vi "AimingBeamCodeTest.vi"() -> ()   [LabVIEW 2024]
doc: "Main VI for FLS imaging system."
uses:
  SubVI/DigitizerConfiguration/FLImDAQ.ctl
  <instrlib>/niScope/Controls/niScope trigger source.ctl
  ConfigFiles/AimingBeamVideoConfig.ctl
  <vilib>/Utility/error.llb/DialogType.ctl
  <vilib>/numeric/Random Number (Range) DBL.vi
  SubVI/GlobalVariables.vi
  <userlib>/_OpenG.lib/file/file.llb/openg_file.lvlib
  <userlib>/_OpenG.lib/time/time.llb/openg_time.lvlib
  <vilib>/Utility/miscctls.llb/LVPointTypeDef.ctl
panel:
  in  "VideoConfig":T1={"DeCon Channel"=enum."1", "Scale Bar"=FALSE, "Scale Low"=10.0, "Scale High"=200.0, "ANSI"=20.0, "Radius"=1.0, "3D?"=FALSE, "Firefly?"=FALSE, "Pentero?"=FALSE}
  out "Lifetime":dbl
  in  "MainLoopExit?":errorcluster
  out "SendLifetime?":bool
  in  "Channel":enum16{"Ch1", "Ch2", "Ch3"}(ring)
  out "Visualization PC video source":T2
  in  "Video Display":bool
  out "ML?":bool
  out "remote address":string
  out "Sync Success?":bool
  out "Disclamer":picture
  out "Calibration #":i8
  out "BG #":i8
  in  "TCP Connect":bool
  out "Help":string
  out "Run":i8 caption="Run #"
  in  "StopButton":bool caption="Stop"
  out "Aquisition Status:":bool
  in  "StartButton":bool caption="Start"
  in  "Video Source":enum32{"Camera", "FrameGrabber"}(radio)
  out "Case #":string
  out "System Hardware Connection Status":T3
  in  "Tab Control":T4(tab)
  out "Communication loop(ms)":u32
  out "FLImDAQ":T5={"Digitizer 1"="", "Digitizer 2"="", "Channel"=enum."Channel 0", "trigger source"="VAL_EXTERNAL", "trigger level"=0.5, "trigger delay"=1.35e-07, "min sample rate"=12500000000.0, "min record length"=2500, "vertical range"=1.0, "vertical offset"=-0.25, "Waveform to Avg"=2000} caption="FLIm DAQ Configuration" {"trigger delay" format="%^#.4e"; "trigger level" min=0.0 max=3.5 step=0.5 format="%.2f"; "vertical offset" format="%.4f"; "vertical range" format="%.2f"; "min sample rate" format="%#.2p"}
  out "data out(communcation loop)":string
  out "syctimer data out":string
  out "State log":string
  in  "Quit":bool
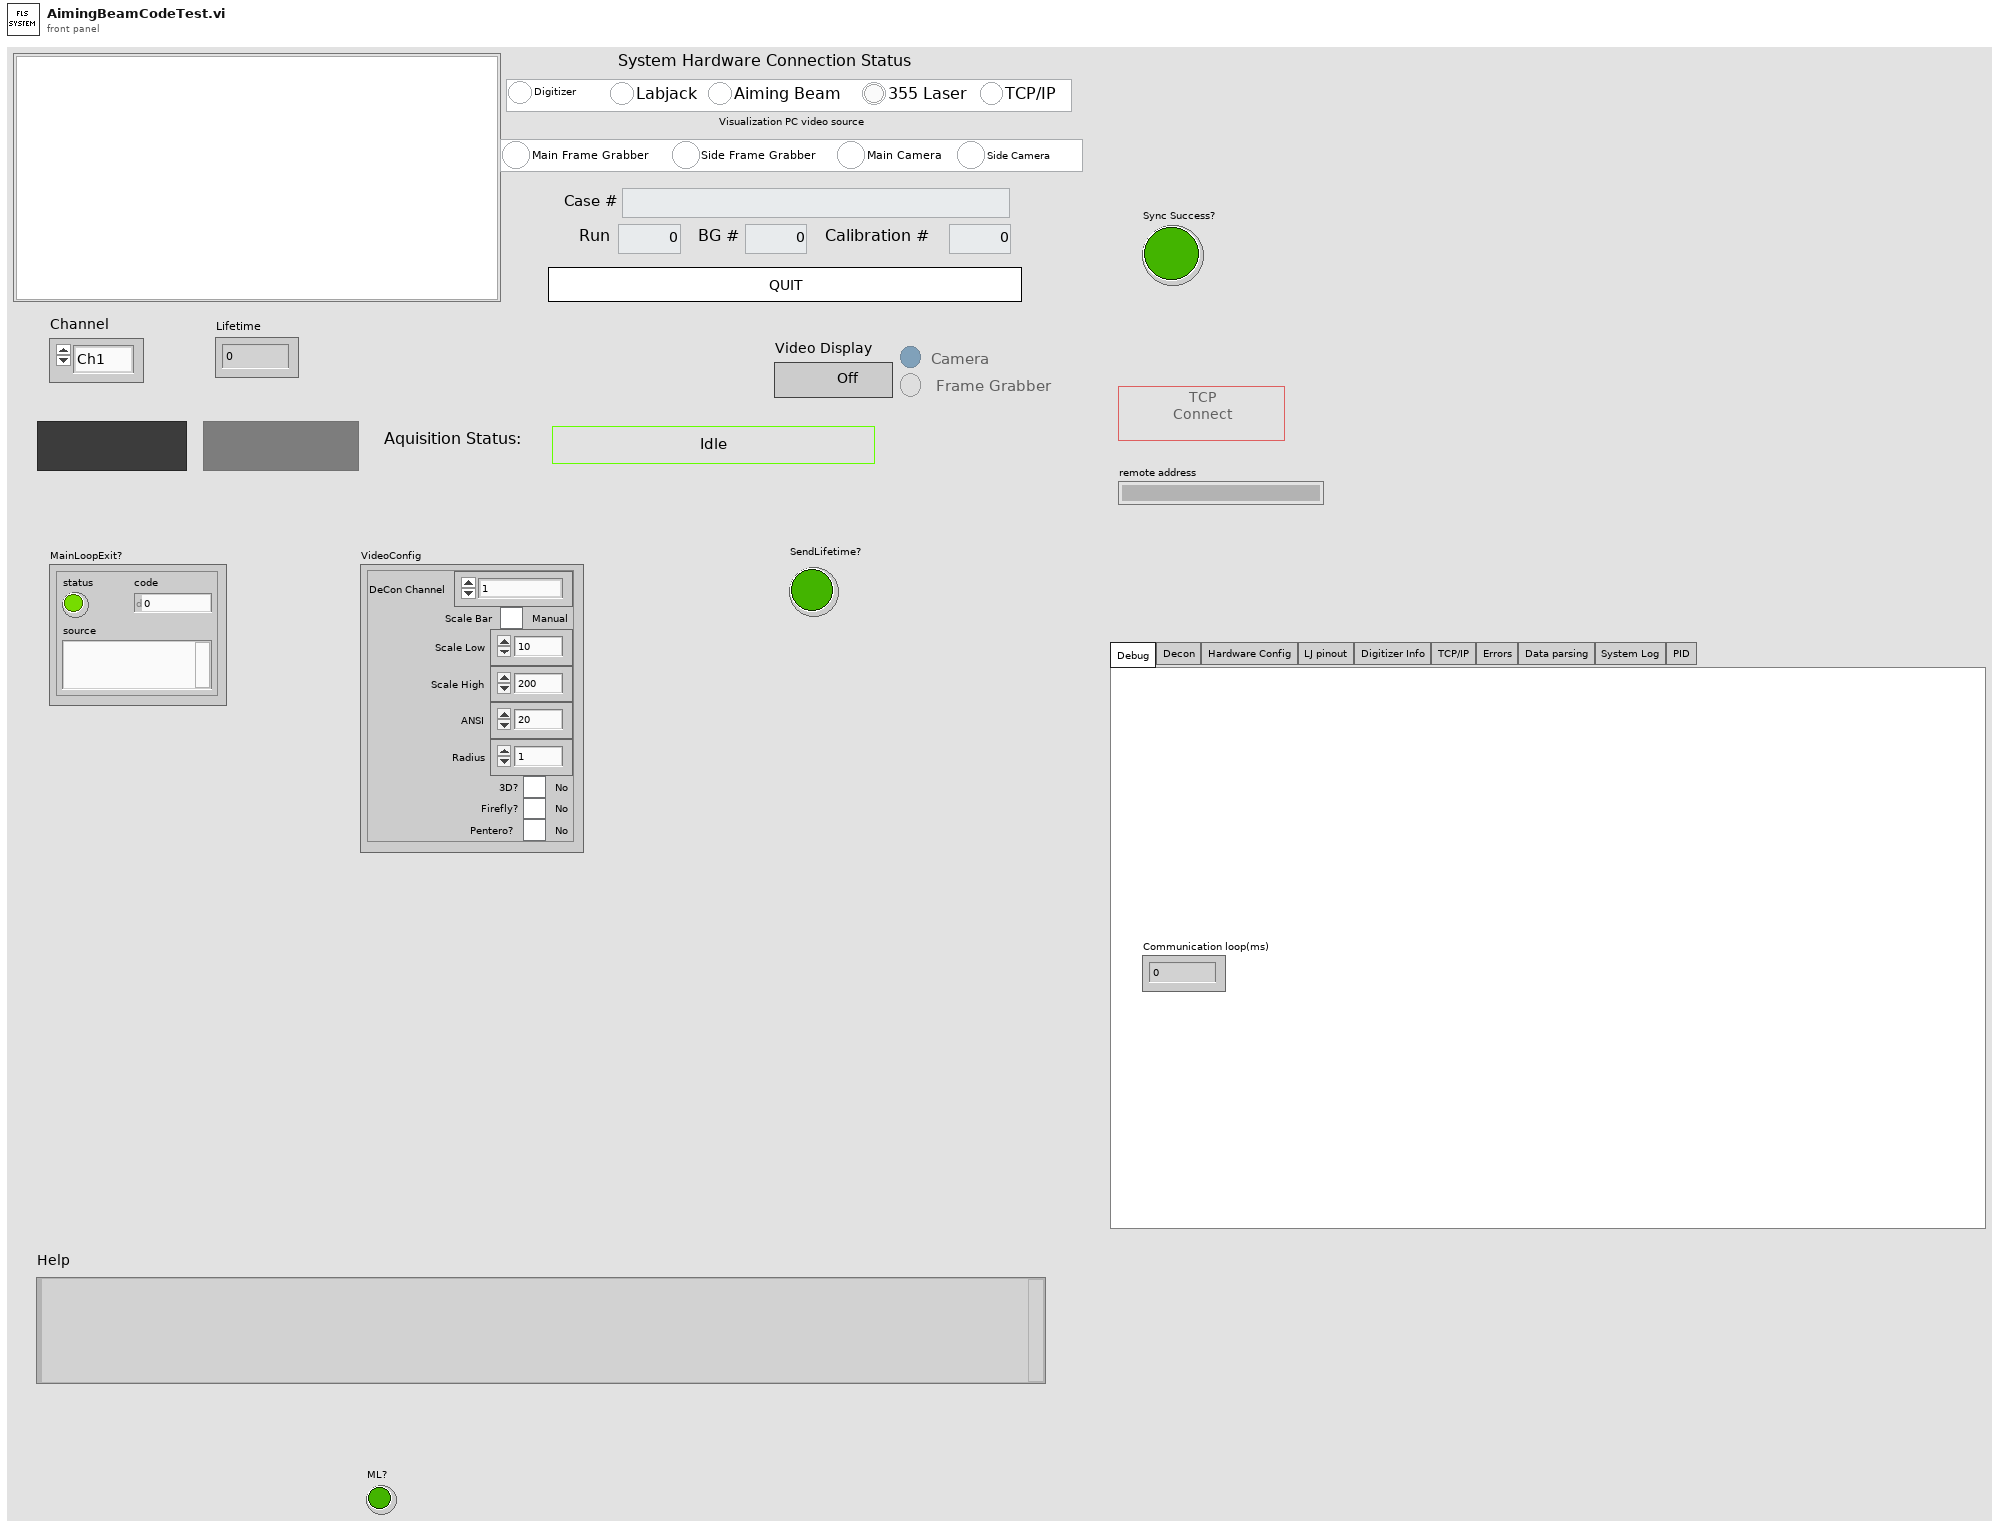
[diagram p1: front panel]
types:
  T1 = typedef "AimingBeamVideoConfig.ctl" = cluster{"DeCon Channel":enum16{"1", "2", "3"}, "Scale Bar":bool, "Scale Low":dbl, "Scale High":dbl, "ANSI":dbl, "Radius":dbl, "3D?":bool, "Firefly?":bool, "Pentero?":bool}
  T2 = cluster{"Main Frame Grabber":bool, "Side Frame Grabber":bool, "Main Camera":bool, "Side Camera":bool}
  T3 = cluster{"Digitizer":bool, "Labjack":bool, "Aiming Beam":bool, "355 Laser":bool, "TCP/IP":bool}
  T4 = enum32{"Debug", "Decon", "Hardware Config", "LJ pinout", "Digitizer Info", "TCP/IP", "Errors", "Data parsing", "System Log", "PID"}
  T5 = typedef "FLImDAQ.ctl" = cluster{"Digitizer 1":refnum<k15>, "Digitizer 2":refnum<k15>, "Channel":enum16{"Channel 0", "Channel 1", "Channel 0&1"}, "trigger source":T6, "trigger level":dbl, "trigger delay":dbl, "min sample rate":dbl, "min record length":i32, "vertical range":dbl, "vertical offset":dbl, "Waveform to Avg":i16}
  T6 = typedef "niScope trigger source.ctl" = string
  T7 = enum8{"Enabled", "Disabled", "Disabled and Grayed Out"}
  T8 = enum16{"open", "replace", "create", "open or create", "replace or create", "replace or create with confirmation"}
  T9 = enum32{"Invalid", "Standard", "Closed", "Hidden", "Minimized", "Maximized"}
  T10 = enum32{"invalid app kind", "Development System", "Run Time System", "Student Edition", "Embedded LabVIEW", "Evaluation", "Custom"}
  T11 = enum16{"Standard", "Buffered", "CRLF", "Immediate"}
  T12 = cluster{"Core":cluster{"Current VI Reference":refnum<vi>, "Close Panel on Exit?":bool}, "System Status":cluster{"Digitizer":bool, "Labjack":bool, "Aiming Beam":bool, "355 Laser":bool, "TCP/IP":bool}, "IDs":cluster{"RunID":i8, "BG ID":i8, "Cali ID":i8}, "CaseID":string, "DefaultPath":path, "Pathes":cluster{"DataPath":path, "BG Path":path, "iRFPath":path, "CaliPath":path}, "FLImDAQ":cluster{"resource name":refnum<k15>, "resource name 2":refnum<k15>, "Channel":enum16{"Channel 0", "Channel 1", "Channel 0&1"}, "trigger source":T6, "trigger level":dbl, "trigger delay":dbl, "min sample rate":dbl, "min record length":i32, "vertical range":dbl, "vertical offset":dbl, "Waveform to Avg":i32}, "SysRunning?":bool, "TCP attempt count":i32, "SlowTimer":u32, "FastTimer":u32, "listener ID":refnum<k5>, "TempPath":path, "VideoConfig":T1, "video source":cluster{"Main Frame Grabber":bool, "Side Frame Grabber":bool, "Main Camera":bool, "Side Camera":bool}, "bothVidSourceAvail":bool}
  T13 = cluster{"DataPath":path, "BG Path":path, "iRFPath":path, "CaliPath":path}
  T14 = cluster{"resource name":refnum<k15>, "resource name 2":refnum<k15>, "Channel":enum16{"Channel 0", "Channel 1", "Channel 0&1"}, "trigger source":T6, "trigger level":dbl, "trigger delay":dbl, "min sample rate":dbl, "min record length":i32, "vertical range":dbl, "vertical offset":dbl, "Waveform to Avg":i32}
  T15 = cluster{"Current VI Reference":refnum<vi>, "Close Panel on Exit?":bool}
  T16 = typedef "DialogType.ctl" = u16
  T17 = typedef "LVBoundsTypeDef.ctl" = cluster{"Width":u32, "Height":u32}
  T18 = typedef "imagedata.ctl" = cluster{"image type":i32, "image depth":i32, "image":u8[], "mask":u8[], "colors":u32[], "Rectangle":cluster{"left":i16, "top":i16, "right":i16, "bottom":i16}}
  T19 = typedef "LVPointTypeDef.ctl" = cluster{"Horizontal":i16, "Vertical":i16}
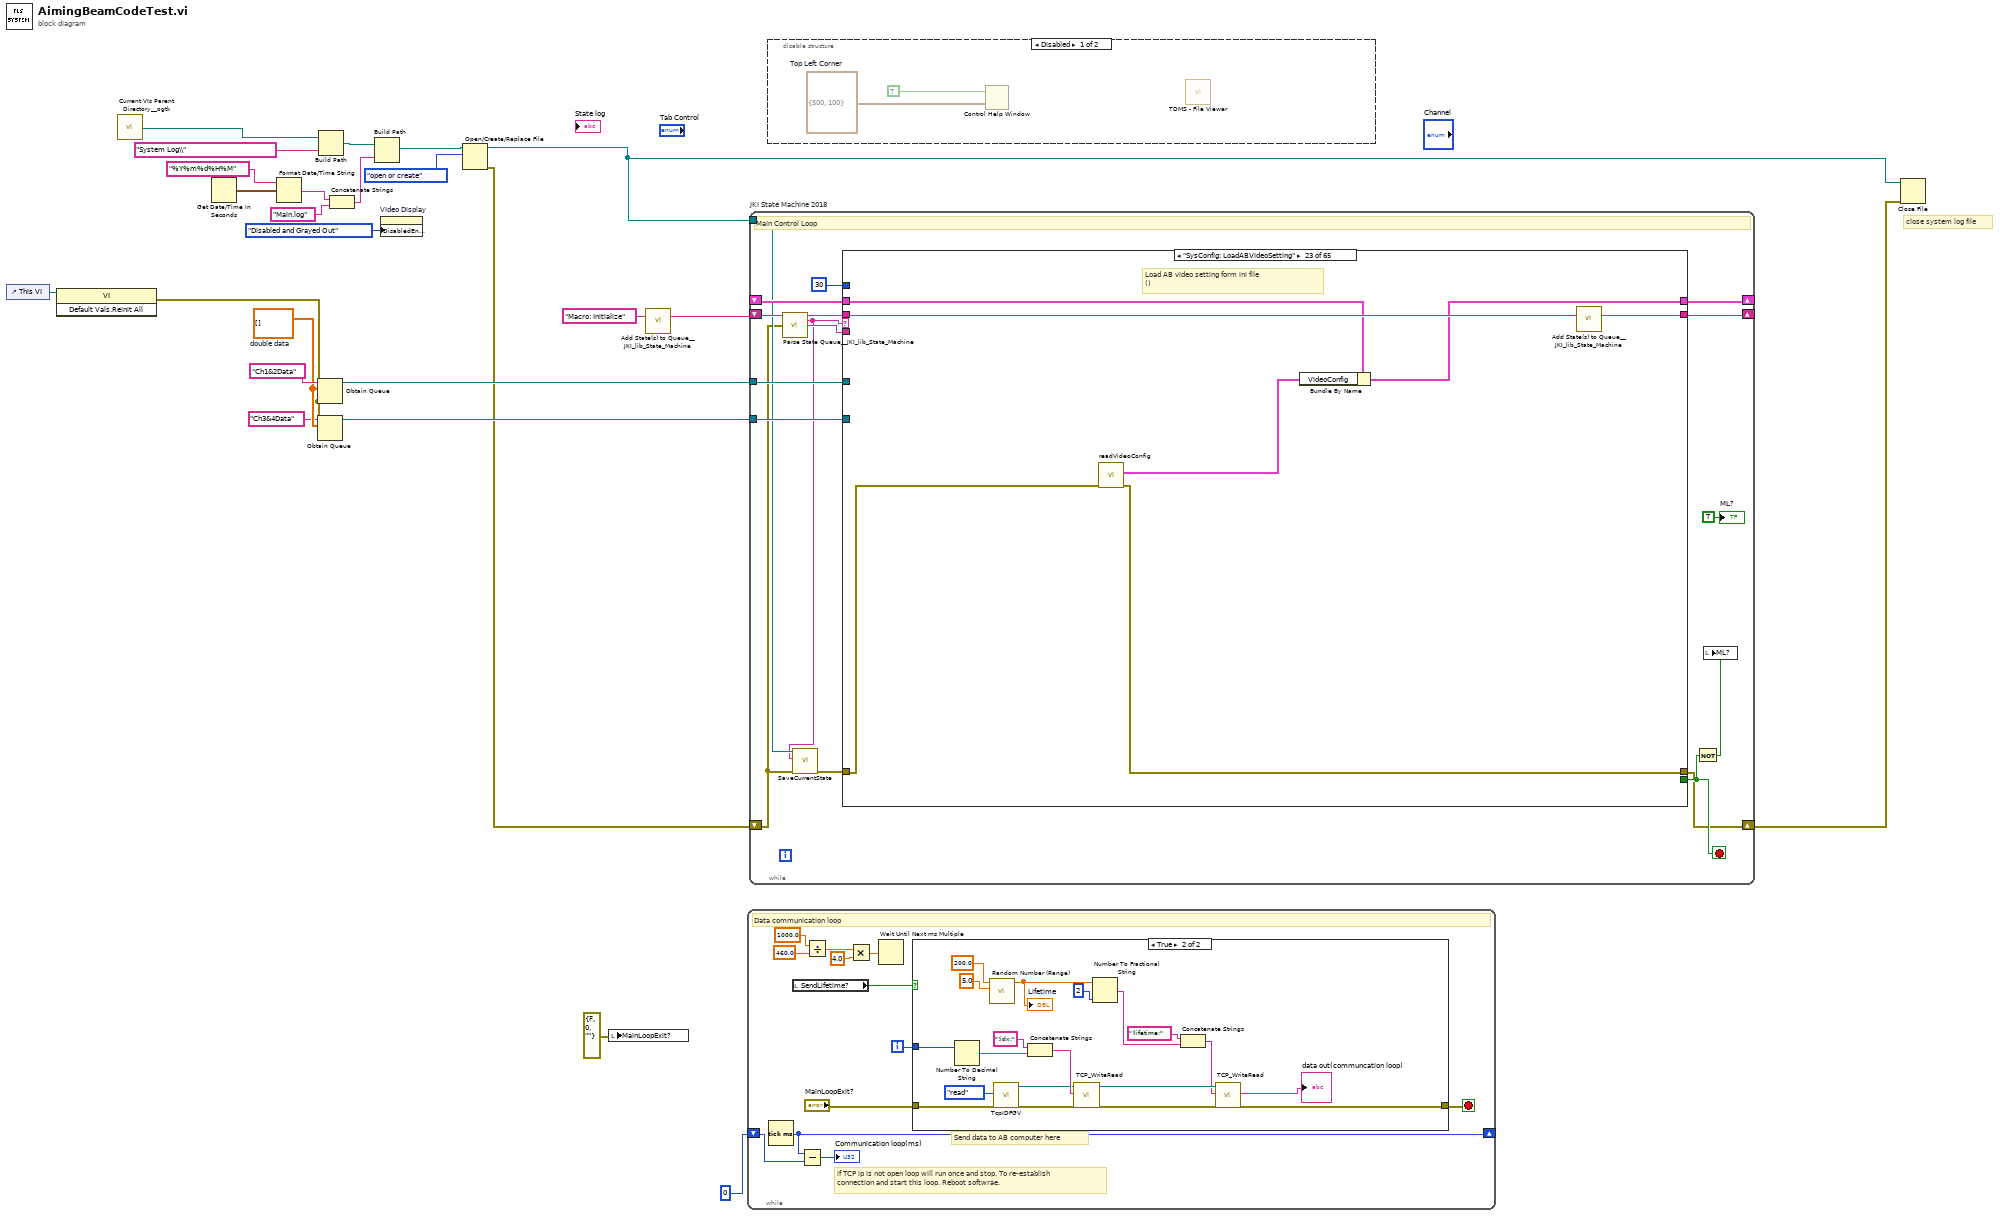
[diagram p0: block diagram]
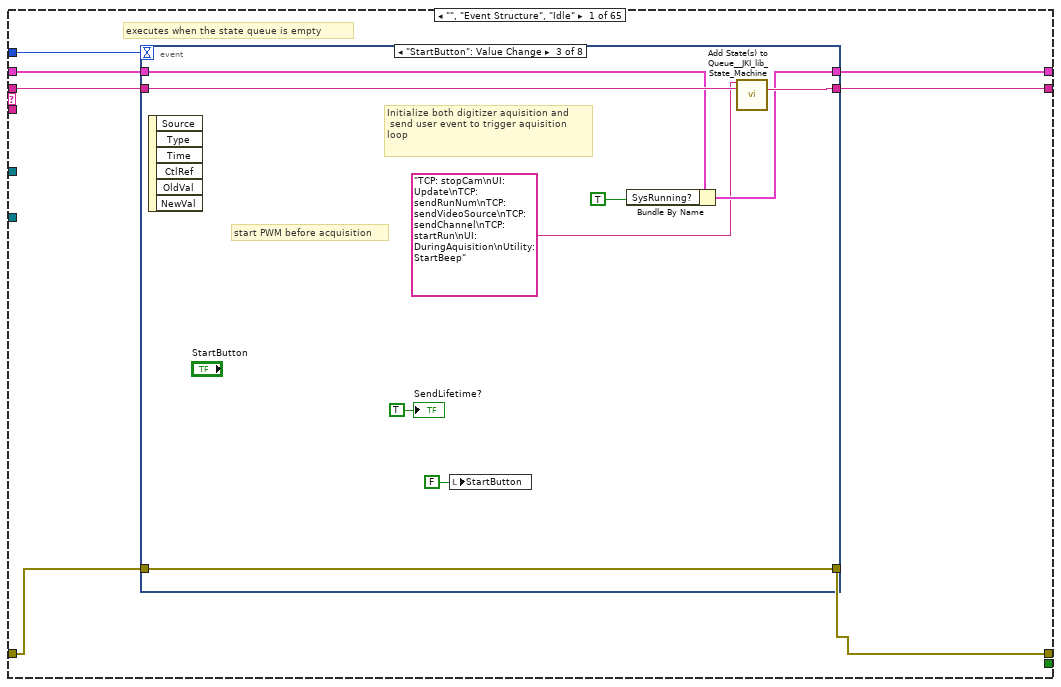
[diagram p2: hidden frame]
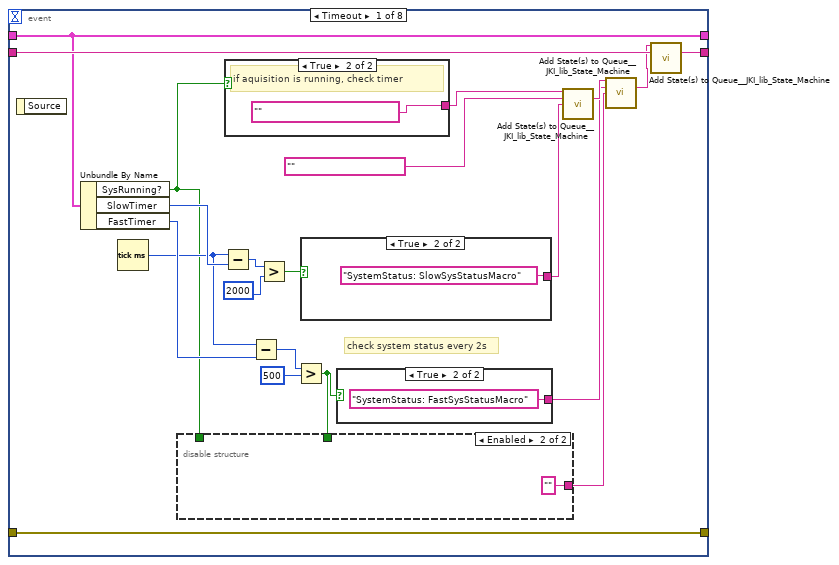
[diagram p3: hidden frame]
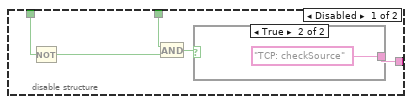
[diagram p4: hidden frame]
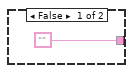
[diagram p5: hidden frame]
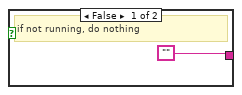
[diagram p6: hidden frame]
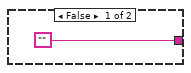
[diagram p7: hidden frame]
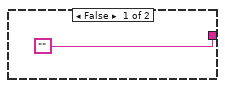
[diagram p8: hidden frame]
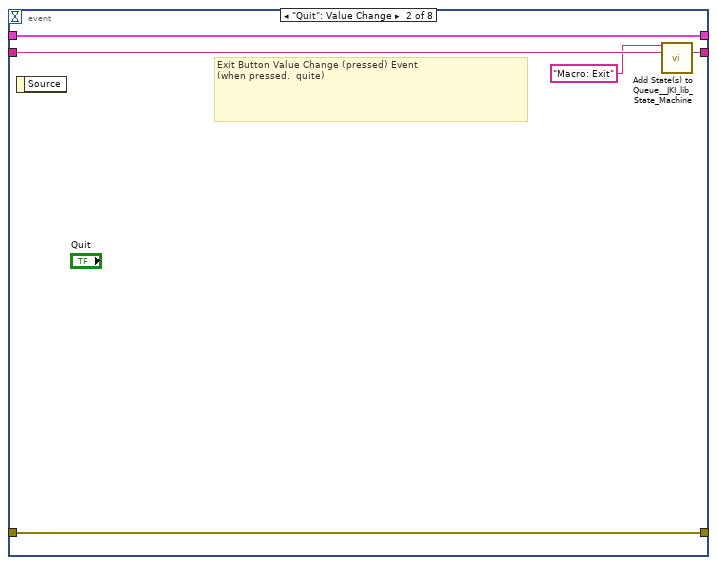
[diagram p9: hidden frame]
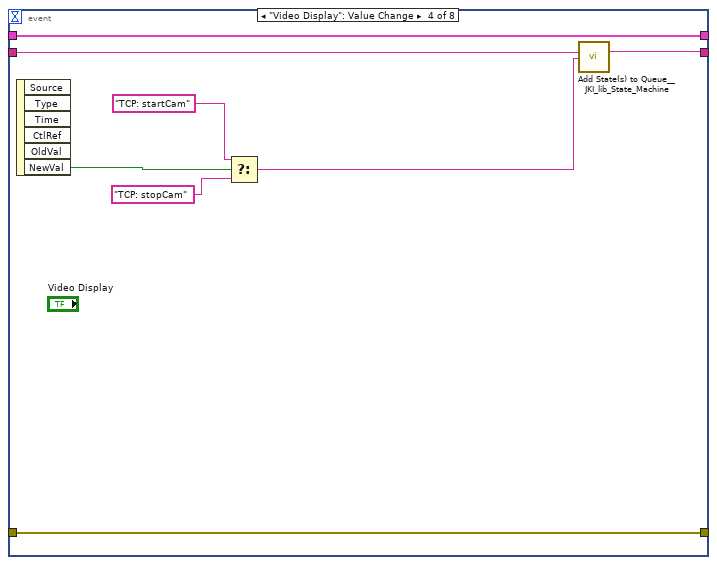
[diagram p10: hidden frame]
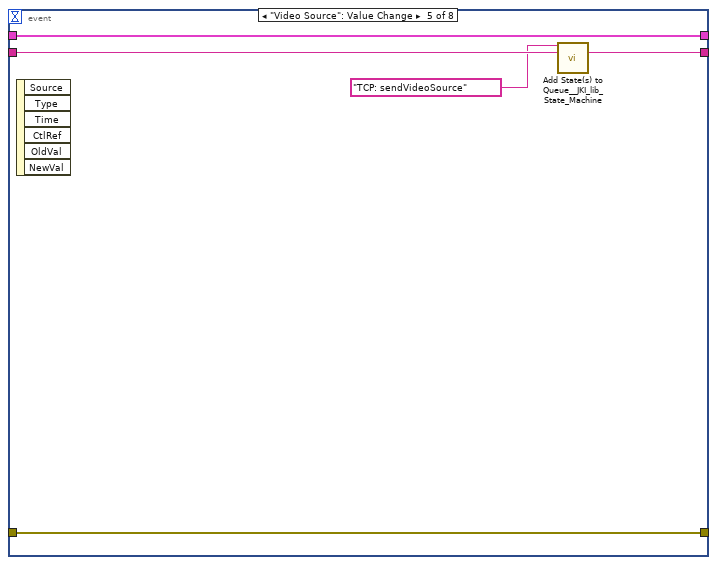
[diagram p11: hidden frame]
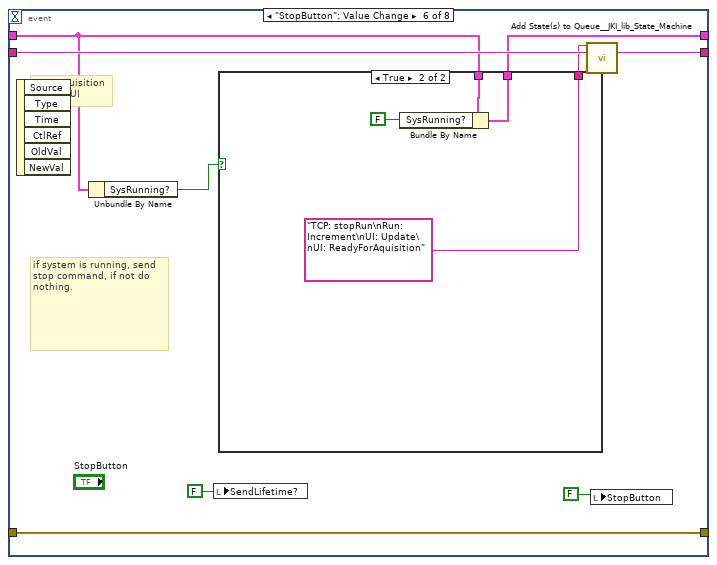
[diagram p12: hidden frame]
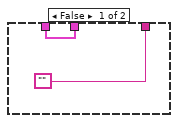
[diagram p13: hidden frame]
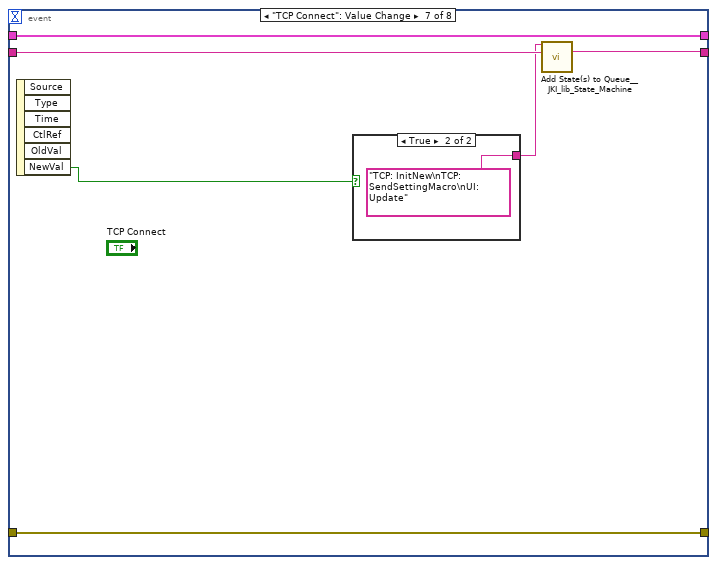
[diagram p14: hidden frame]
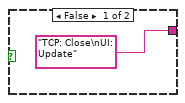
[diagram p15: hidden frame]
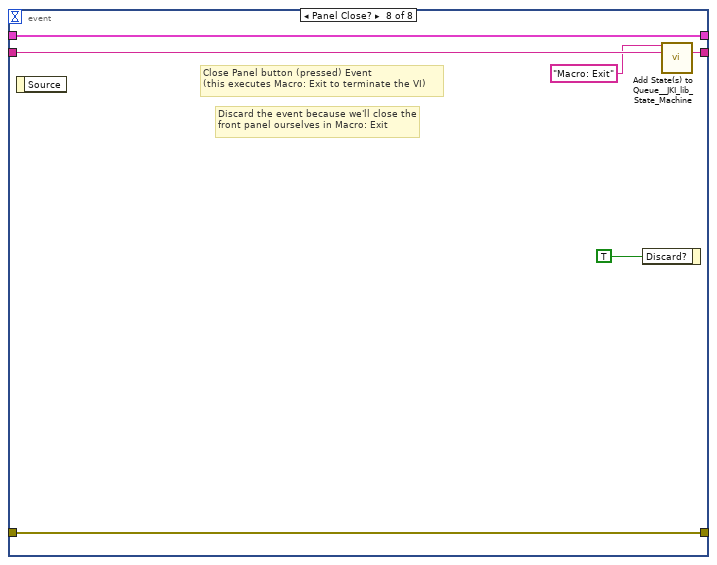
[diagram p16: hidden frame]
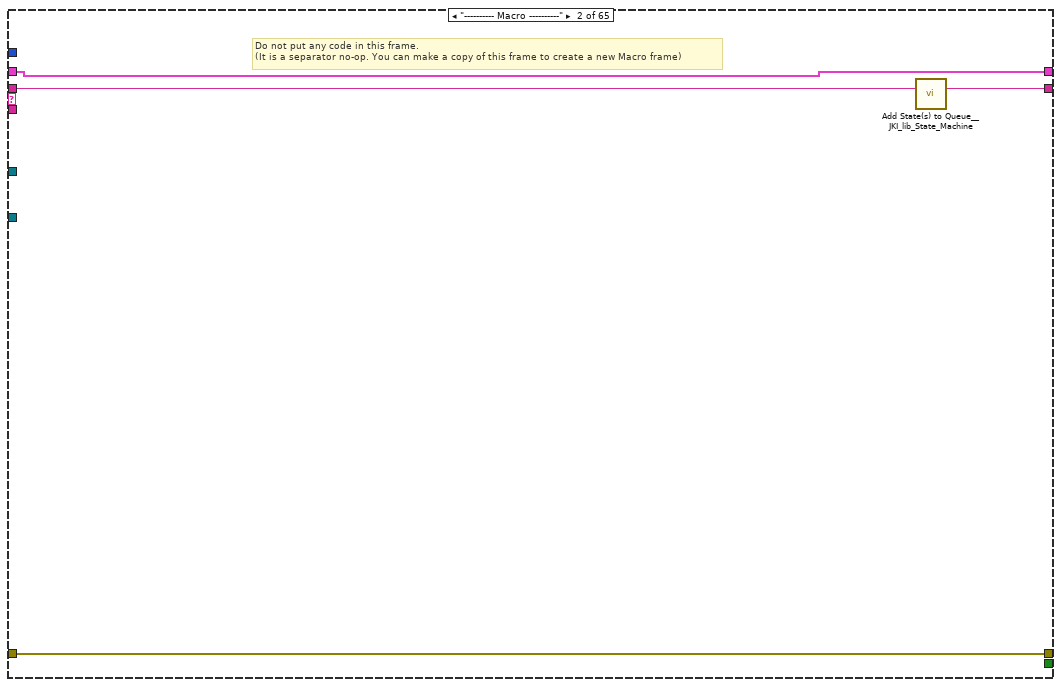
[diagram p17: hidden frame]
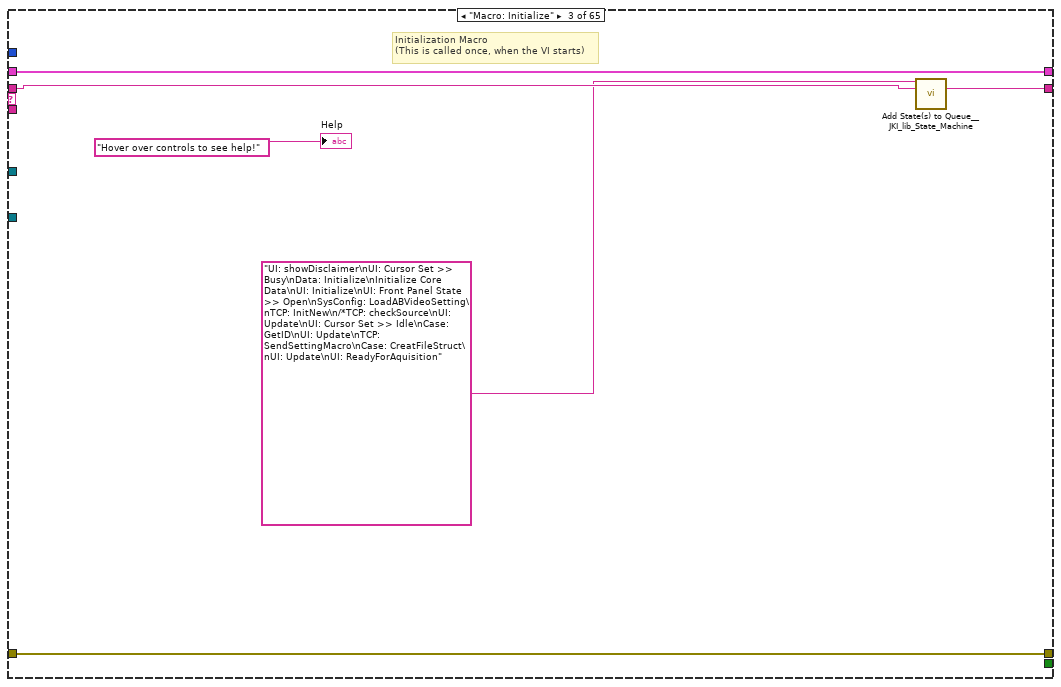
[diagram p18: hidden frame]
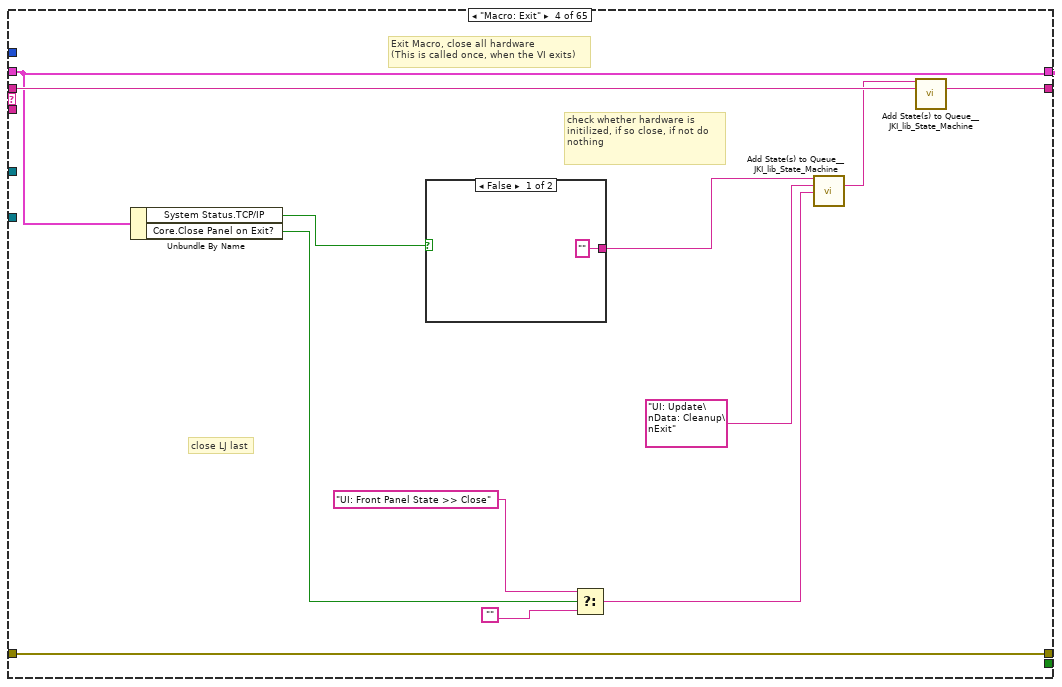
[diagram p19: hidden frame]
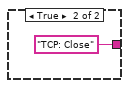
[diagram p20: hidden frame]
diagram:
  w21 = dbl[][] []  # double data
  # "close system log file"
  n1 = control-ref of="This VI"() -> (w23:refnum<vi>)
  n2 = invoke on="Invoke Node" class="VI" method="Default Vals.Reinit All"(reference=w23) -> (error out=w6:errorcluster)  [unwired: 2 in, 2 out]
  n3 = call <userlib>:"Current VIs Parent Directory__ogtk.vi"() -> ("Parent Directory (+ Relative)"=w16:path)  [unwired: 5 in]
  n4 = Get Date/Time In Seconds() -> (seconds since 1Jan1904=w14:timestamp)
  n5 = Format Date/Time String(time format string (%c)="%Y%m%d%H%M", seconds (now)=w14) -> (date/time string=w11:string)  [unwired: 1 in]
  n6 = Obtain Queue(name (unnamed)="Ch3&4Data", element data type=w21, error in (no error)=w6) -> (queue out=w18:refnum<queue>)  [unwired: 2 in, 2 out]
  n7 = Obtain Queue(name (unnamed)="Ch1&2Data", element data type=w21, error in (no error)=w6) -> (queue out=w19:refnum<queue>)  [unwired: 2 in, 2 out]
  n8 = Build Path(base path=w16, name or relative path="System Log\\") -> (appended path=w7:path)
  n9 = Concatenate Strings(w11, "Main.log" ("string")) -> (w9:string)
  n10 = Build Path(base path=w7, name or relative path=w9) -> (appended path=w12:path)
  n11 = property on="Video Display" class="Bool (strict)"("DisabledEnum"=T7."Disabled and Grayed Out" ("Disabled")) -> ()  [unwired: 2 in, 2 out]
  n12 = Open/Create/Replace File(file path (use dialog)=w12, operation (0:open)=T8."open or create") -> (refnum out=w4:refnum<file>, error out=w5:errorcluster)  [unwired: 4 in, 1 out]
  n13 = local write "MainLoopExit?"(errorcluster {"status"=FALSE, "code"=0, "source"=""} ("MainLoopExit?")) -> ()
  n14 = call <vilib>:"Add State(s) to Queue__JKI_lib_State_Machine.vi"("State(s) in (\"\")"="Macro: Initialize") -> ("States Out"=w25:string)  [unwired: 14 in]
  n15 = while {
    shift-right: [w35] -> _
    shift-left: u32 0 -> [w36]
    i -> [w33]
    stop <- w34 stop-if-true
    # "Send data to AB computer here"
    # "if TCP ip is not open loop will run once and stop. To re-establish connection and start this loop. Reboot softwrae."
    # "Data communication loop"
    n16 = Tick Count (ms)() -> (millisecond timer value=w35:u32)
    n17 = local read "SendLifetime?"() -> (w31:bool)
    n18 = Subtract(x=w35, y=w36) -> (x-y=→"Communication loop(ms)":u32)
    n19 = Divide(x=1000.0, y=460.0) -> (x/y=w28:dbl)
    n20 = Multiply(x=w28, y=4.0) -> (x*y=w26:dbl)
    n21 = Wait Until Next ms Multiple(millisecond multiple=w26) -> ()  [unwired: 1 out]
    n22 = case shown="True" w31 {
      tunnel: w33 -> [_ w48]
      tunnel: "MainLoopExit?" -> [w38 w45]
      tunnel: [w38 w42] -> w34
      frame False {
      }
      frame True {
        n23 = Number To Decimal String(number=w48) -> (decimal integer string=w56:string)  [unwired: 1 in]
        n24 = call-poly <vilib>:"Random Number (Range).vi"("lower bound (0)"=5.0 ("upper bound (100)"), "upper bound (100)"=200.0) -> ("number"=w39:dbl)  [unwired: 9 in]
        "Lifetime" <- w39
        n25 = call "TcpIDFGV.vi"("Error In"=w45, "action"=enum16{"write", "read"}."read") -> ("Error Out"=w44:errorcluster, "connection ID out"=w54:refnum<k5>)  [unwired: 8 in]
        n26 = Concatenate Strings("!idx:", w56) -> (w57:string)
        n27 = call "TCP_WriteRead.vi"("error in (no error)"=w44, "data in"=w57, "connectin ID in"=w54) -> ("error out"=w43:errorcluster, "connectin ID out"=w55:refnum<k5>)  [unwired: 4 in, 1 out]
        n28 = Number To Fractional String(number=w39, precision (6)=i16 2) -> (F-format string=w47:string)  [unwired: 2 in]
        n29 = Concatenate Strings("!lifetime:", w47) -> (w53:string)
        n30 = call "TCP_WriteRead.vi"("error in (no error)"=w43, "data in"=w53, "connectin ID in"=w55) -> ("error out"=w42:errorcluster, "data out"=→"data out(communcation loop)":string)  [unwired: 4 in, 1 out]
      }
    }
  }
  n31 = while "JKI State Machine 2018" {
    shift-right: [w70] -> _
    shift-left: _ -> [w69]
    shift-right: [w58] -> w3
    shift-left: w5 -> [w60]
    shift-right: [w71] -> _
    shift-left: w25 -> [w72]
    tunnel: w19 -> [w67]
    tunnel: w18 -> [w66]
    tunnel: w4 -> [w62]
    stop <- w65 stop-if-true
    # "Main Control Loop"
    n32 = call <vilib>:"Parse State Queue__JKI_lib_State_Machine.vi"("State Queue"=w72, "Error In (no error)"=w60) -> ("Remaining States"=w74:string, "Current State"=w61:string, "Arguments"=w73:string)  [unwired: 11 in]
    n33 = call "SaveCurrentState.vi"("error in (no error)"=w60, "Current State"=w61, "Byte Stream File in"=w62) -> ("error out"=w59:errorcluster)  [unwired: 8 in]
    n34 = case shown="\"SysConfig: LoadABVideoSetting\"" w61 {
      selector: w61 -> [_ _ _ _ _ _ _ _ w231 _ _ _ _ _ _ _ _ _ _ _ _ _ _ _ _ _ _ _ _ _ _ _ _ _ _ _ _ _ _ _ _ _ _ _ _ _ _ _ _ _ _ _ _ _ _ _ _ _ _ _ _ _ _ _ _]
      tunnel: w74 -> [w81 w176 w182 w194 w200 w220 w226 w230 w235 w261 w268 w291 w295 w307 w325 w350 w375 w412 w416 w423 w430 w434 w441 w445 w451 w457 w461 w465 w482 w491 w501 w515 w521 w532 w601 w608 w612 w625 w629 w633 w637 w664 w701 w751 w796 w840 w850 w867 w886 w899 w918 w939 w955 w975 w998 w1016 w1033 w1050 w1067 w1080 w1093 w1110 w1123 w1139 w1153]
      tunnel: w73 -> [_ _ _ _ _ _ _ _ _ _ _ _ _ _ _ _ _ _ _ _ _ _ _ _ _ _ _ _ _ _ _ _ w516 w526 _ _ _ w622 _ _ _ _ _ _ _ _ _ _ _ _ _ _ _ _ _ _ _ _ _ _ _ _ _ _ _]
      tunnel: w69 -> [w79 w173 w179 w191 w197 _ w221 w227 w233 w254 w265 w289 w292 w296 w316 w341 w367 w408 w413 w418 w425 w431 w436 w442 w446 w452 w458 w464 w479 w486 w496 w512 w519 w528 w598 w605 w609 w619 w626 w630 w634 w645 w695 w746 w793 w837 w847 w863 w882 w895 w916 w934 w951 w971 w994 w1012 w1029 w1046 w1063 w1076 w1089 w1106 w1119 w1135 w1150]
      tunnel: [w78 w174 w180 w192 w198 w218 w222 w228 w237 w258 errorcluster {"status"=FALSE, "code"=0, "source"=""} ("error out") w288 w293 w305 w323 w348 w366 w410 w414 w421 w428 w432 w439 w443 w449 w455 w459 w463 w480 w488 w498 w513 w517 w529 w599 w606 w610 w623 w627 w631 w635 w647 w689 w747 w794 w838 w846 w865 w884 w897 w907 w936 w953 w973 w996 w1014 w1031 w1048 w1065 w1078 w1091 w1108 w1121 w1136 w1151] -> w58
      tunnel: w59 -> [w77 w174 w180 w192 w198 w218 w223 w228 w236 w258 w262 w288 w293 w305 w323 w348 w365 w410 w414 w421 w428 w432 w438 w443 w449 w455 w459 w463 w480 w488 w498 w513 w518 w530 w599 w606 w610 w623 w627 w631 w635 w662 _ w748 w794 w838 w845 w864 w883 w896 w912 w935 w952 w972 w995 w1013 w1030 w1047 w1064 w1077 w1090 w1107 w1120 w1133 w1151]
      tunnel: [w80 w175 w181 w193 w199 w219 w225 w229 w234 w260 w267 w290 w294 w306 w324 w349 w374 w411 w415 w422 w429 w433 w440 w444 w450 w456 w460 w465 w481 w490 w500 w514 w520 w531 w600 w607 w611 w624 w628 w632 w636 w663 w700 w750 w795 w839 w849 w866 w885 w898 w917 w938 w954 w974 w997 w1015 w1032 w1049 w1066 w1079 w1092 w1109 w1122 w1138 w1152] -> w71
      tunnel: [_ _ _ _ _ _ _ _ _ _ _ TRUE _ _ _ _ _ _ _ _ _ _ _ _ _ _ _ _ _ _ _ _ _ _ _ _ _ _ _ _ _ _ _ _ _ _ _ _ _ _ _ _ _ _ _ _ _ _ _ _ _ _ _ _ _] -> w65
      tunnel: [w76 w173 w179 w191 w197 w207 w221 w227 w233 w259 w265 w289 w292 w297 w317 w342 w368 w409 w413 w419 w426 w431 w437 w442 w447 w453 w458 w464 w479 w486 w496 w512 w519 w528 w598 w605 w609 w619 w626 w630 w634 w646 w699 w745 w793 w837 w847 w863 w882 w895 w916 w934 w951 w971 w994 w1012 w1029 w1046 w1063 w1076 w1089 w1106 w1119 w1137 w1150] -> w70
      tunnel: 30 ("Timeout") -> [w75 _ _ _ _ _ _ _ _ _ _ _ _ _ _ _ _ _ _ _ _ _ _ _ _ _ _ _ _ _ _ _ _ _ _ _ _ _ _ _ _ _ _ _ _ _ _ _ _ _ _ _ _ _ _ _ _ _ _ _ _ _ _ _ _]
      tunnel: w67 -> [_ _ _ _ _ _ _ _ _ _ _ _ _ _ _ _ _ _ _ _ _ _ _ _ _ _ _ _ _ _ _ _ _ _ _ _ _ _ _ _ _ _ _ _ _ _ _ _ _ _ _ _ _ _ _ _ _ _ _ _ _ _ _ _ _]
      tunnel: w66 -> [_ _ _ _ _ _ _ _ _ _ _ _ _ _ _ _ _ _ _ _ _ _ _ _ _ _ _ _ _ _ _ _ _ _ _ _ _ _ _ _ _ _ _ _ _ _ _ _ _ _ _ _ _ _ _ _ _ _ _ _ _ _ _ _ _]
      frame "", "Event Structure", "Idle" {
        # "executes when the state queue is empty"
        n35 = event shown="[2] \"StartButton\": Value Change" {
          selector: _ -> [_ _ _ _ _ _ _ _]
          dyn-events: _ -> [_ _ _ _ _ _ _ _]
          timeout: w75 -> [_ _ _ _ _ _ _ _]
          tunnel: w81 -> [w101 w121 w129 w135 w141 w151 w162 w172]
          tunnel: [w102 w120 w130 w134 w140 w152 w161 w171] -> w80
          tunnel: w79 -> [w85 w117 w126 w137 w142 w146 w163 w169]
          tunnel: [w100 w119 w123 w138 w143 w150 w164 w170] -> w78
          tunnel: w77 -> [w100 w119 w123 w138 w143 w150 w164 w170]
          tunnel: [w85 w117 w127 w137 w142 w147 w163 w169] -> w76
          event Timeout {
            # "check system status every 2s"
            n36 = event-data() -> ()  [unwired: 1 in, 1 out]
            n37 = Unbundle By Name(w85) -> ("SysRunning?"=w83:bool, "SlowTimer"=w99:u32, "FastTimer"=w93:u32)
            n38 = Tick Count (ms)() -> (millisecond timer value=w86:u32)
            n39 = Subtract(x=w86, y=w99) -> (x-y=w96:u32)
            n40 = case shown="True" w83 {
              tunnel: ["" "" ("State(s) in Front (\"\")")] -> w91
              frame False {
                # "if not running, do nothing"
              }
              frame True {
                # "if aquisition is running, check timer"
              }
            }
            n41 = Subtract(x=w86, y=w93) -> (x-y=w94:u32)
            n42 = Greater?(x=w96, y=u32 2000) -> (0:w97:bool)
            n43 = Greater?(x=w94, y=u32 500) -> (0:w84:bool)
            n44 = disable-structure shown="Enabled" {
              disable-tunnel: w84 -> [w107 _]
              disable-tunnel: w83 -> [w106 _]
              disable-tunnel: [w103 "" ("State(s) at Back (\"\")")] -> w82
              frame Disabled {
                n45 = Not(x=w106) -> (.not. x?=w105:bool)
                n46 = And(x=w107, y=w105) -> (x .and. y?=w104:bool)
                n47 = case shown="True" w104 {
                  tunnel: ["" ("Empty String Constant") "TCP: checkSource" ("State(s) in Front (\"\")")] -> w103
                  frame False {
                  }
                  frame True {
                  }
                }
              }
              frame Enabled {
              }
            }
            n48 = case shown="True" w97 {
              tunnel: ["" ("Empty String Constant") "SystemStatus: SlowSysStatusMacro" ("State(s) in Front (\"\")")] -> w89
              frame False {
              }
              frame True {
              }
            }
            n49 = case shown="True" w84 {
              tunnel: ["" ("Empty String Constant") "SystemStatus: FastSysStatusMacro" ("State(s) in Front (\"\")")] -> w87
              frame False {
              }
              frame True {
              }
            }
            n50 = call <vilib>:"Add State(s) to Queue__JKI_lib_State_Machine.vi"("State(s) in Front (\"\")"=w91, "State(s) in (\"\")"="" ("State(s) in Front (\"\")"), "State(s) at Back (\"\")"=w89) -> ("States Out"=w88:string)  [unwired: 12 in]
            n51 = call <vilib>:"Add State(s) to Queue__JKI_lib_State_Machine.vi"("State(s) in Front (\"\")"=w88, "State(s) in (\"\")"=w87, "State(s) at Back (\"\")"=w82) -> ("States Out"=w92:string)  [unwired: 12 in]
            n52 = call <vilib>:"Add State(s) to Queue__JKI_lib_State_Machine.vi"("State(s) in Front (\"\")"=w92, "State(s) in (\"\")"=w101) -> ("States Out"=w102:string)  [unwired: 13 in]
          }
          event "Quit": Value Change {
            # "Exit Button Value Change (pressed) Event\n(when pressed.  quite)"
            n53 = event-data() -> ()  [unwired: 1 in, 1 out]
            n54 = call <vilib>:"Add State(s) to Queue__JKI_lib_State_Machine.vi"("State(s) in Front (\"\")"="Macro: Exit", "State(s) in (\"\")"=w121) -> ("States Out"=w120:string)  [unwired: 13 in]
          }
          event "StartButton": Value Change {
            # "start PWM before acquisition"
            # "Initialize both digitizer aquisition and\n send user event to trigger aquisition loop"
            n55 = event-data() -> ()  [unwired: 1 in, 6 out]
            n56 = local write "StartButton"(FALSE ("StartButton")) -> ()
            n57 = Bundle By Name(cluster=w126, "SysRunning?"=TRUE) -> (w127:T12)
            n58 = call <vilib>:"Add State(s) to Queue__JKI_lib_State_Machine.vi"("State(s) in Front (\"\")"="TCP: stopCam\nUI: Update\nTCP: sendRunNum\nTCP: sendVideoSource\nTCP: sendChannel\nTCP: startRun\nUI: DuringAquisition\nUtility: StartBeep", "State(s) in (\"\")"=w129) -> ("States Out"=w130:string)  [unwired: 13 in]
            "SendLifetime?" <- TRUE ("SendLifetime?")
          }
          event "Video Display": Value Change {
            n59 = event-data() -> ("NewVal"=w136:bool)  [unwired: 1 in, 5 out]
            n60 = Select(t="TCP: startCam", s=w136, f="TCP: stopCam") -> (s? t:f=w133:string)
            n61 = call <vilib>:"Add State(s) to Queue__JKI_lib_State_Machine.vi"("State(s) in (\"\")"=w135, "State(s) at Back (\"\")"=w133) -> ("States Out"=w134:string)  [unwired: 13 in]
          }
          event "Video Source": Value Change {
            n62 = event-data() -> ()  [unwired: 1 in, 6 out]
            n63 = call <vilib>:"Add State(s) to Queue__JKI_lib_State_Machine.vi"("State(s) in Front (\"\")"="TCP: sendVideoSource" ("State(s) in Front (\"\")"), "State(s) in (\"\")"=w141) -> ("States Out"=w140:string)  [unwired: 13 in]
          }
          event "StopButton": Value Change {
            # "if system is running, send stop command, if not do nothing."
            # "stop aquisition\nupdate UI"
            n64 = event-data() -> ()  [unwired: 1 in, 6 out]
            n65 = Unbundle By Name(w146) -> ("SysRunning?"=w148:bool)
            n66 = local write "SendLifetime?"(FALSE ("SendLifetime?")) -> ()
            n67 = case shown="True" w148 {
              tunnel: ["" ("Empty String Constant") "TCP: stopRun\nRun: Increment\nUI: Update\nUI: ReadyForAquisition"] -> w149
              tunnel: w146 -> [w153 w157]
              tunnel: [w153 w156] -> w147
              frame False {
              }
              frame True {
                n68 = Bundle By Name(cluster=w157, "SysRunning?"=FALSE) -> (w156:T12)
              }
            }
            n69 = call <vilib>:"Add State(s) to Queue__JKI_lib_State_Machine.vi"("State(s) in Front (\"\")"=w149, "State(s) in (\"\")"=w151) -> ("States Out"=w152:string)  [unwired: 13 in]
            n70 = local write "StopButton"(FALSE ("StopButton")) -> ()
          }
          event "TCP Connect": Value Change {
            n71 = event-data() -> ("NewVal"=w159:bool)  [unwired: 1 in, 5 out]
            n72 = case shown="True" w159 {
              tunnel: ["TCP: Close\nUI: Update" ("State(s) in Front (\"\")") "TCP: InitNew\nTCP: SendSettingMacro\nUI: Update" ("State(s) in Front (\"\")")] -> w160
              frame False {
              }
              frame True {
              }
            }
            n73 = call <vilib>:"Add State(s) to Queue__JKI_lib_State_Machine.vi"("State(s) in Front (\"\")"=w160, "State(s) in (\"\")"=w162) -> ("States Out"=w161:string)  [unwired: 13 in]
          }
          event Panel Close? {
            # "Discard the event because we'll close the front panel ourselves in Macro: Exit"
            # "Close Panel button (pressed) Event\n(this executes Macro: Exit to terminate the VI)"
            n74 = event-data() -> ()  [unwired: 1 in, 1 out]
            n75 = event-data ("Event Filter Node")("Discard?"=TRUE) -> ()  [unwired: 1 in, 1 out]
            n76 = call <vilib>:"Add State(s) to Queue__JKI_lib_State_Machine.vi"("State(s) in Front (\"\")"="Macro: Exit", "State(s) in (\"\")"=w172) -> ("States Out"=w171:string)  [unwired: 13 in]
          }
        }
      }
      frame "---------- Macro ----------" {
        # "Do not put any code in this frame.\n(It is a separator no-op. You can make a copy of this frame to create a new Macro frame)"
        n77 = call <vilib>:"Add State(s) to Queue__JKI_lib_State_Machine.vi"("State(s) in (\"\")"=w176) -> ("States Out"=w175:string)  [unwired: 14 in]
      }
      frame "Macro: Initialize" {
        # "Initialization Macro\n(This is called once, when the VI starts)"
        n78 = call <vilib>:"Add State(s) to Queue__JKI_lib_State_Machine.vi"("State(s) in Front (\"\")"="UI: showDisclaimer\nUI: Cursor Set >> Busy\nData: Initialize\nInitialize Core Data\nUI: Initialize\nUI: Front Panel State >> Open\nSysConfig: LoadABVideoSetting\nTCP: InitNew\n/*TCP: checkSource\nUI: Update\nUI: Cursor Set >> Idle\nCase: GetID\nUI: Update\nTCP: SendSettingMacro\nCase: CreatFileStruct\nUI: Update\nUI: ReadyForAquisition" ("State(s) in Front (\"\")"), "State(s) in (\"\")"=w182) -> ("States Out"=w181:string)  [unwired: 13 in]
        "Help" <- "Hover over controls to see help!" ("Help")
      }
      frame "Macro: Exit" {
        # "close LJ last"
        # "check whether hardware is initilized, if so close, if not do nothing"
        # "Exit Macro, close all hardware\n(This is called once, when the VI exits)"
        n79 = Unbundle By Name(w191) -> ("System Status.TCP/IP"=w184:bool, "Core.Close Panel on Exit?"=w187:bool)
        n80 = case shown="False" w184 {
          tunnel: ["" "TCP: Close"] -> w183
          frame False {
          }
          frame True {
          }
        }
        n81 = Select(t="UI: Front Panel State >> Close", s=w187, f="" ("Empty String Constant")) -> (s? t:f=w185:string)
        n82 = call <vilib>:"Add State(s) to Queue__JKI_lib_State_Machine.vi"("State(s) in Front (\"\")"=w183, "State(s) in (\"\")"="UI: Update\nData: Cleanup\nExit", "State(s) at Back (\"\")"=w185) -> ("States Out"=w188:string)  [unwired: 12 in]
        n83 = call <vilib>:"Add State(s) to Queue__JKI_lib_State_Machine.vi"("State(s) in Front (\"\")"=w188, "State(s) in (\"\")"=w194) -> ("States Out"=w193:string)  [unwired: 13 in]
      }
      frame "---------- Data ----------" {
        # "Do not put any code in this frame.\n(It is a separator no-op. You can make a copy of this frame to create a new Data frame)"
        n84 = call <vilib>:"Add State(s) to Queue__JKI_lib_State_Machine.vi"("State(s) in (\"\")"=w200) -> ("States Out"=w199:string)  [unwired: 14 in]
      }
      frame "Data: Initialize" {
        w202 = FALSE  # bothVidSourceAvail
        w203 = T2 {"Main Frame Grabber"=FALSE, "Side Frame Grabber"=FALSE, "Main Camera"=FALSE, "Side Camera"=FALSE}  # video source
        w204 = cluster{"RunID":i8, "BG ID":i8, "Cali ID":i8} {"RunID"=1, "BG ID"=1, "Cali ID"=1}  # IDs
        w205 = path ""  # TempPath
        w206 = T13 {"DataPath"=path "", "BG Path"=path "", "iRFPath"=path "", "CaliPath"=path ""}  # Pathes
        w209 = u32 0  # FastTimer
        w210 = u32 0  # SlowTimer
        w212 = T3 {"Digitizer"=FALSE, "Labjack"=FALSE, "Aiming Beam"=FALSE, "355 Laser"=FALSE, "TCP/IP"=FALSE}  # System Status
        w213 = 0  # TCP attempt count
        w214 = T14 {"resource name"="", "resource name 2"="", "Channel"=enum."Channel 0", "trigger source"="VAL_EXTERNAL", "trigger level"=0.5, "trigger delay"=1.35e-07, "min sample rate"=12500000000.0, "min record length"=2500, "vertical range"=1.0, "vertical offset"=-0.25, "Waveform to Avg"=2000}  # FLImDAQ
        w215 = FALSE  # SysRunning?
        w211 = path ""  # DefaultPath
        w216 = ""  # CaseID
        w217 = T15 {"Current VI Reference"=refnum, "Close Panel on Exit?"=FALSE}  # Core
        # "Initialize the shift-register data, here.\n(data names are defined by what you wire into the bundle function)"
        n85 = Bundle("Core"=w217, "System Status"=w212, "IDs"=w204, "CaseID"=w216, "DefaultPath"=w211, "Pathes"=w206, "FLImDAQ"=w214, "SysRunning?"=w215, "TCP attempt count"=w213, "SlowTimer"=w210, "FastTimer"=w209, "listener ID"=refnum<k5> refnum, "TempPath"=w205, "VideoConfig"="VideoConfig", "video source"=w203, "bothVidSourceAvail"=w202) -> (w207:T12)  [unwired: 1 in]
        n86 = call <vilib>:"Add State(s) to Queue__JKI_lib_State_Machine.vi"("State(s) in (\"\")"=w220) -> ("States Out"=w219:string)  [unwired: 14 in]
      }
      frame "Data: Cleanup" {
        # "Cleanup any data and references, here.\n(this is called automatically, by the Macro: Exit)"
        n87 = Unbundle By Name(w221) -> ("Core.Current VI Reference"=w224:refnum<vi>)
        n88 = Close Reference(reference=w224, error in (no error)=w223) -> (error out=w222:errorcluster)
        n89 = call <vilib>:"Add State(s) to Queue__JKI_lib_State_Machine.vi"("State(s) in (\"\")"=w226) -> ("States Out"=w225:string)  [unwired: 14 in]
      }
      frame "---------- Core ----------" {
        # "Do not put any code in this frame.\n(it is a separator no-op)"
        n90 = call <vilib>:"Add State(s) to Queue__JKI_lib_State_Machine.vi"("State(s) in (\"\")"=w230) -> ("States Out"=w229:string)  [unwired: 14 in]
      }
      frame Default {
        w240 = 42 items=["No error", "Argument error", "Memory is full", "Out of zone", "End of file", "File already open", "Generic file I/O error", "File not found", "File permission error", "Disk is full", "Duplicate path", "Too many files open", "System feature not enabled", "Resource file not found", "Cannot add resource", "Resource not found", "Image not found", "Image memory error", "Pen does not exist", "Config type invalid", "Config token not found", "Config parse error", "Config memory error", "Bad external code format", "Bad external code offset", "External code not present", "Null window", "Destroy window error", "Null menu", "Print aborted", "Bad print record", "Print driver error", "Windows error during printing", "Memory error during printing", "Print dialog error", "Generic print error", "Invalid device refnum", "Device not found", "Device parameter error", "Device unit error", "Cannot open device", "Device call aborted", "Generic error", "Cancelled by user", "Object ID too low", "Object ID too high", "Object not in heap", "Unknown heap", "Unknown object (invalid DefProc)", "Unknown object (DefProc not in table)", "Message out of range", "Invalid (null) method", "Unknown message", "Manager call not supported", "Bad address", "Network operation in progress", "Network operation timed out", "Connection is busy", "Network attribute not supported", "Network error", "Address in use", "System out of memory", "Connection aborted", "Connection refused", "Not connected", "Already connected", "Connection closed", "Initialization error (interapplication manager)", "Bad occurrence", "Wait on unbound occurrence handler", "Occurrence queue overflow", "Datalog type conflict", "Unused", "Unrecognized type (interapplication manager)", "Memory corrupt", "Failed to make temporary DLL", "Old CIN version", "Drag socket not found", "Failed to load drop-object", "Failed to register OLE object", "Failed to release OLE object", "Format specifier type mismatch", "Unknown format specifier", "Too few format specifiers", "Too many format specifiers", "Scan failed", "Newer CIN version", "Error converting to variant", "Runtime menu error", "Password tampered", "Variant attribute not found", "Incompatible variant data type", "Event data is not available", "Event Store is not present", "Occurrence is not found", "Event Queue is not created", "Event info is not available", "Refnum passed is NULL", "Error retrieving Class GUID", "Error retrieving CoClass GUID", "Error retrieving TypeLib GUID.", "Bad built application magic bytes.", "Specific driver is different from the specific driver associated with the Logical Name.", "There is no session opened to the class driver.", "Max Error", "MAX - Error with config objects", "MAX - Error loading configuration", "MAX - Group not supported"]
        # "Current State"
        # "Do not delete, rename, or modify this frame.\n(this is used to capture unhandled states and typos)"
        # "Handle mistyped state name (developer tool)"
        n91 = Format Into String(format string="Software Exception: Unhandled State \"%s\"." ("message"), error in=w236, w231) -> (resulting string=w239:string, error out=w238:errorcluster)  [unwired: 1 in]
        n92 = call <vilib>:"Error Cluster From Error Code.vi"("show call chain? (False)"=TRUE, "error in (no error)"=w238, "error message (\"\")"=w239, "error code (0)"=w240) -> ("error out"=w237:errorcluster)  [unwired: 5 in]
        n93 = call <vilib>:"Add State(s) to Queue__JKI_lib_State_Machine.vi"("State(s) in (\"\")"=w235) -> ("States Out"=w234:string)  [unwired: 14 in]
      }
      frame "Initialize Core Data" {
        # "Build default path based on the location of project"
        # "Do not delete, rename, or modify this frame.\n(this is used to determine panel behavior on exit)"
        # "originally closed?"
        # "exe?"
        # "If panel starts closed or is an EXE, then close it when we exit"
        n94 = call <vilib>:"Application Directory.vi"() -> ("Application Directory"=w244:path)
        n95 = property on="Property Node" class="App"() -> ("App.Kind"=w257:T10)  [unwired: 2 in, 2 out]
        n96 = property on="Property Node" class="VI"() -> ("FP.State"=w251:T9)  [unwired: 2 in, 2 out]
        n97 = control-ref of="Current VI Reference"() -> (w252:refnum<vi>)
        n98 = Equal?(x=w251, y=T9."Closed" ("Front Panel Window:State")) -> (x = y?=w249:bool)
        n99 = Equal?(x=w257, y=T10."Run Time System" ("Application:Kind")) -> (x = y?=w255:bool)
        n100 = Build Path(base path=w244, name or relative path="Data") -> (appended path=w247:path)
        n101 = Build Path(base path=w244, name or relative path="SystemTemp") -> (appended path=w245:path)
        n102 = Build Path(base path=w244, name or relative path="SystemCalibrationFile") -> (appended path=w242:path)
        n103 = Or(x=w249, y=w255) -> (x .or. y?=w253:bool)
        n104 = Bundle By Name(cluster=w254, "Core.Current VI Reference"=w252, "Core.Close Panel on Exit?"=w253, "DefaultPath"=w247, "TempPath"=w245, "Pathes.CaliPath"=w242) -> (w259:T12)
        n105 = call <vilib>:"Add State(s) to Queue__JKI_lib_State_Machine.vi"("State(s) in (\"\")"=w261) -> ("States Out"=w260:string)  [unwired: 14 in]
      }
      frame "Error Handler" {
        # "Unhandled Error -- Display it"
        # "Handle any errors here.\nYou can also output any states to clean-up after errors occur"
        # "Clear error"
        n106 = Unbundle By Name(w262) -> ("code"=w264:i32)
        n107 = case shown="5001" w264 {
          tunnel: ["Macro: Exit" w273 w279] -> w263
          tunnel: w262 -> [w269 _ _]
          frame Default {
            w271 = T16 1 items=["no dialog", "OK message", "continue or stop message", "OK message + warnings", "continue/stop + warnings"] ("type of dialog (OK msg:1)")
            n108 = call <vilib>:"General Error Handler.vi"("type of dialog (OK msg:1)"=w271, "error in (no error)"=w269) -> ()  [unwired: 9 in, 5 out]
          }
          frame 5002 {
            n109 = Two Button Dialog(message="Laser interlock open! Please close interlock and try again! ", 1:"Safely Shutdown" ("F button name (\"Cancel\")"), 2:"OK" ("T button name (\"OK\")")) -> (T button?=w274:bool)
            n110 = case shown="True" w274 {
              tunnel: ["Macro: Exit" ""] -> w273
              frame False {
              }
              frame True {
              }
            }
          }
          frame 5001 {
            n111 = Two Button Dialog(message="Unable to connect to imaging computer, do you want to run data aquisiton alone? ", 1:"No" ("F button name (\"Cancel\")"), 2:"Yes" ("T button name (\"OK\")")) -> (T button?=w280:bool)
            n112 = case shown="False" w280 {
              tunnel: ["Macro: Exit" "" ("Empty String Constant")] -> w279
              frame False {
              }
              frame True {
              }
            }
          }
        }
        n113 = call <vilib>:"Add State(s) to Queue__JKI_lib_State_Machine.vi"("State(s) in Front (\"\")"=w263, "State(s) in (\"\")"=w268) -> ("States Out"=w267:string)  [unwired: 13 in]
      }
      frame "Exit" {
        # "Do not put any code in this frame.\n(No errors that occur here will be handled.)"
        n114 = local write "MainLoopExit?"(errorcluster {"status"=TRUE, "code"=0, "source"=""} ("MainLoopExit?")) -> ()
        n115 = call <vilib>:"Add State(s) to Queue__JKI_lib_State_Machine.vi"("State(s) in (\"\")"=w291) -> ("States Out"=w290:string)  [unwired: 14 in]
      }
      frame "---------- Case ----------" {
        # "Template Separator\n(You can make a copy of, or modify, this frame)"
        n116 = call <vilib>:"Add State(s) to Queue__JKI_lib_State_Machine.vi"("State(s) in (\"\")"=w295) -> ("States Out"=w294:string)  [unwired: 14 in]
      }
      frame "Case: getCaliID" {
        # "Get Calibration file #\n(You can make a copy of, or modify, this frame)"
        n117 = Unbundle By Name(w296) -> ("Pathes.CaliPath"=w299:path)
        n118 = call <vilib>:"Recursive File List.vi"("pattern"="*.tdms", "Treat LLBs as Folders?"=FALSE, "Folder Path"=w299) -> ("All Files in Dir"=w304:path[])  [unwired: 4 in, 4 out]
        n119 = for {
          tunnel: w304 -> [w313] mode=indexing
          tunnel: [w312] -> w303 mode=indexing
          tunnel: "Calibration" -> [w309]
          n120 = Strip Path(path=w313) -> (name=w310:string)  [unwired: 1 out]
          n121 = Search and Replace String(input string=w310, search string=w309) -> (result string=w308:string)  [unwired: 6 in, 3 out]
          n122 = Scan From String(format string="%d" ("string"), input string=w308) -> (output 1=w312:i32)  [unwired: 3 in, 3 out]
        }
        n123 = Array Max & Min(array=w303) -> (max value=w302:i32)  [unwired: 3 out]
        n124 = Bundle By Name(cluster=w296, "IDs.Cali ID"=w302) -> (w297:T12)
        n125 = call <vilib>:"Add State(s) to Queue__JKI_lib_State_Machine.vi"("State(s) in (\"\")"=w307) -> ("States Out"=w306:string)  [unwired: 14 in]
      }
      frame "Case: getBGID" {
        # "Get background #\n(You can make a copy of, or modify, this frame)"
        n126 = Unbundle By Name(w316) -> ("Pathes.BG Path"=w321:path)
        n127 = call <vilib>:"Recursive File List.vi"("pattern"="*.tdms", "Treat LLBs as Folders?"=FALSE, "Folder Path"=w321) -> ("All Files in Dir"=w319:path[])  [unwired: 4 in, 4 out]
        n128 = for {
          tunnel: w319 -> [w335] mode=indexing
          tunnel: "Background" ("name or relative path") -> [w333]
          shift-right: [w326] -> w314
          shift-left: 0 -> [w330]
          n129 = Strip Path(path=w335) -> (name=w334:string)  [unwired: 1 out]
          n130 = Search and Replace String(input string=w334, search string=w333) -> (number of replacements=w332:i32)  [unwired: 6 in, 3 out]
          n131 = Greater Than 0?(x=w332) -> (x > 0?=w331:bool)
          n132 = Select(t=1, s=w331, f=0) -> (s? t:f=w329:i32)
          n133 = Add(x=w329, y=w330) -> (x+y=w326:i32)
        }
        n134 = Bundle By Name(cluster=w316, "IDs.BG ID"=w314) -> (w317:T12)
        n135 = call <vilib>:"Add State(s) to Queue__JKI_lib_State_Machine.vi"("State(s) in (\"\")"=w325) -> ("States Out"=w324:string)  [unwired: 14 in]
      }
      frame "Case: getRunID" {
        # "Check folder for run ID\n(You can make a copy of, or modify, this frame)"
        n136 = Unbundle By Name(w341) -> ("Pathes.DataPath"=w340:path, "CaseID"=w336:string)
        n137 = Build Array("Background" ("name or relative path"), "Calibration") -> (w347:string[])
        n138 = call <vilib>:"Recursive File List.vi"("Folders to Exclude"=w347, "pattern"="*.tdms", "Treat LLBs as Folders?"=FALSE, "Folder Path"=w340) -> ("All Files in Dir"=w337:path[])  [unwired: 3 in, 4 out]
        n139 = for {
          tunnel: w337 -> [w356] mode=indexing
          tunnel: [w355] -> w343 mode=indexing
          tunnel: w336 -> [w352]
          n140 = Strip Path(path=w356) -> (name=w353:string)  [unwired: 1 out]
          n141 = Search and Replace String(input string=w353, search string=w352) -> (result string=w351:string)  [unwired: 6 in, 3 out]
          n142 = Scan From String(format string="_%d" ("string"), input string=w351) -> (output 1=w355:i32)  [unwired: 3 in, 3 out]
        }
        n143 = Array Max & Min(array=w343) -> (max value=w344:i32)  [unwired: 3 out]
        n144 = Bundle By Name(cluster=w341, "IDs.RunID"=w344) -> (w342:T12)
        n145 = call <vilib>:"Add State(s) to Queue__JKI_lib_State_Machine.vi"("State(s) in (\"\")"=w350) -> ("States Out"=w349:string)  [unwired: 14 in]
      }
      frame "Case: CreatFileStruct" {
        # "Creat case file structure"
        n146 = Unbundle By Name(w367) -> ("DefaultPath"=w373:path, "CaseID"=w359:string)
        n147 = Build Path(base path=w373, name or relative path=w359) -> (appended path=w372:path)
        n148 = call <vilib>:"Check if File or Folder Exists.vi"("error in (no error)"=w365, "path"=w372) -> ("error out"=w369:errorcluster, "file or folder exists?"=w371:bool, "dup path"=w370:path)  [unwired: 7 in]
        n149 = case shown="True" w371 {
          tunnel: w370 -> [w390 w398]
          tunnel: w369 -> [w388 w393]
          tunnel: [w382 w398] -> w364
          tunnel: [w386 w400] -> w366
          tunnel: [u32 0 u32 0] -> w358
          tunnel: [w384 w403] -> w363
          tunnel: "Background" ("name or relative path") -> [w383 w395]
          tunnel: "Calibration" -> [w381 w394]
          tunnel: [w377 w396] -> w360
          tunnel: w359 -> [_ _]
          tunnel: ["" ("Empty String Constant") "Case: getRunID\nCase: getBGID\nCase: getCaliID\nUI: Update"] -> w357
          frame False {
            # "Folder not exist. Creat folders."
            n150 = Create Folder(path (use dialog)=w390, error in=w388) -> (created path=w382:path, error out=w379:errorcluster)  [unwired: 1 in, 1 out]
            n151 = Build Path(base path=w382, name or relative path=w381) -> (appended path=w380:path)
            n152 = Build Path(base path=w382, name or relative path=w383) -> (appended path=w389:path)
            n153 = Create Folder(path (use dialog)=w389, error in=w379) -> (created path=w384:path, error out=w385:errorcluster)  [unwired: 1 in, 1 out]
            n154 = Create Folder(path (use dialog)=w380, error in=w379) -> (created path=w377:path, error out=w378:errorcluster)  [unwired: 1 in, 1 out]
            n155 = Merge Errors(w385, w378) -> (w386:errorcluster)
          }
          frame True {
            # "Folder exsit, check file #"
            n156 = Build Path(base path=w398, name or relative path=w394) -> (appended path=w399:path)
            n157 = Build Path(base path=w398, name or relative path=w395) -> (appended path=w404:path)
            n158 = call <vilib>:"Check if File or Folder Exists.vi"("path"=w399) -> ("file or folder exists?"=w397:bool, "dup path"=w396:path)  [unwired: 8 in, 1 out]
            n159 = call <vilib>:"Check if File or Folder Exists.vi"("path"=w404) -> ("file or folder exists?"=w402:bool, "dup path"=w403:path)  [unwired: 8 in, 1 out]
            n160 = And(x=w402, y=w397) -> (x .and. y?=w401:bool)
            n161 = case shown="False" w401 {
              tunnel: w393 -> [_ w406]
              tunnel: [errorcluster {"status"=TRUE, "code"=5003, "source"="File structure error."} ("error out") w406] -> w400
              frame False {
              }
              frame True {
              }
            }
          }
        }
        n162 = Bundle By Name(cluster=w367, "Pathes.DataPath"=w364, "Pathes.BG Path"=w363, "Pathes.CaliPath"=w360, "IDs.RunID"=w358, "IDs.BG ID"=w358, "IDs.Cali ID"=w358) -> (w368:T12)
        n163 = call <vilib>:"Add State(s) to Queue__JKI_lib_State_Machine.vi"("State(s) in Front (\"\")"=w357, "State(s) in (\"\")"=w375) -> ("States Out"=w374:string)  [unwired: 13 in]
      }
      frame "Case: GetID" {
        # "Template Separator\n(You can make a copy of, or modify, this frame)"
        n164 = call "set_subjectID.vi"() -> ("subject_id"=w407:string)  [unwired: 10 in]
        n165 = Bundle By Name(cluster=w408, "CaseID"=w407) -> (w409:T12)
        n166 = call <vilib>:"Add State(s) to Queue__JKI_lib_State_Machine.vi"("State(s) in (\"\")"=w412) -> ("States Out"=w411:string)  [unwired: 14 in]
      }
      frame "---------- Run ----------" {
        # "Template Separator\n(You can make a copy of, or modify, this frame)"
        n167 = call <vilib>:"Add State(s) to Queue__JKI_lib_State_Machine.vi"("State(s) in (\"\")"=w416) -> ("States Out"=w415:string)  [unwired: 14 in]
      }
      frame "Run: Increment" {
        # "Increase Run# by 1"
        n168 = Unbundle By Name(w418) -> ("IDs.RunID"=w420:i8)
        n169 = Increment(x=w420) -> (x+1=w417:i8)
        n170 = Bundle By Name(cluster=w418, "IDs.RunID"=w417) -> (w419:T12)
        n171 = call <vilib>:"Add State(s) to Queue__JKI_lib_State_Machine.vi"("State(s) in (\"\")"=w423) -> ("States Out"=w422:string)  [unwired: 14 in]
      }
      frame "Run: Decrement" {
        # "Increase Run# by 1"
        n172 = Unbundle By Name(w425) -> ("IDs.RunID"=w427:i8)
        n173 = Decrement(x=w427) -> (x-1=w424:i8)
        n174 = Bundle By Name(cluster=w425, "IDs.RunID"=w424) -> (w426:T12)
        n175 = call <vilib>:"Add State(s) to Queue__JKI_lib_State_Machine.vi"("State(s) in (\"\")"=w430) -> ("States Out"=w429:string)  [unwired: 14 in]
      }
      frame "---------- SysConfig ----------" {
        # "Template Separator\n(You can make a copy of, or modify, this frame)"
        n176 = call <vilib>:"Add State(s) to Queue__JKI_lib_State_Machine.vi"("State(s) in (\"\")"=w434) -> ("States Out"=w433:string)  [unwired: 14 in]
      }
      frame "SysConfig: LoadABVideoSetting" {
        # "Load AB video setting form ini file\n()"
        n177 = call "readVideoConfig.vi"("error in (no error)"=w438) -> ("error out"=w439:errorcluster, "Aiming Beam Config"=w435:T1)  [unwired: 8 in, 1 out]
        n178 = Bundle By Name(cluster=w436, "VideoConfig"=w435) -> (w437:T12)
        n179 = call <vilib>:"Add State(s) to Queue__JKI_lib_State_Machine.vi"("State(s) in (\"\")"=w441) -> ("States Out"=w440:string)  [unwired: 14 in]
      }
      frame "---------- SystemStatus ----------" {
        # "Template Separator\n(You can make a copy of, or modify, this frame)"
        n180 = call <vilib>:"Add State(s) to Queue__JKI_lib_State_Machine.vi"("State(s) in (\"\")"=w445) -> ("States Out"=w444:string)  [unwired: 14 in]
      }
      frame "SystemStatus: SlowSysStatusMacro" {
        # "store system check time"
        # "Template Separator\n(You can make a copy of, or modify, this frame)"
        n181 = Tick Count (ms)() -> (millisecond timer value=w448:u32)
        n182 = Bundle By Name(cluster=w446, "SlowTimer"=w448) -> (w447:T12)
        n183 = call <vilib>:"Add State(s) to Queue__JKI_lib_State_Machine.vi"("State(s) in (\"\")"=w451) -> ("States Out"=w450:string)  [unwired: 14 in]
      }
      frame "SystemStatus: FastSysStatusMacro" {
        # "store system check time"
        # "Template Separator\n(You can make a copy of, or modify, this frame)"
        n184 = Tick Count (ms)() -> (millisecond timer value=w454:u32)
        n185 = Bundle By Name(cluster=w452, "FastTimer"=w454) -> (w453:T12)
        n186 = call <vilib>:"Add State(s) to Queue__JKI_lib_State_Machine.vi"("State(s) in (\"\")"=w457) -> ("States Out"=w456:string)  [unwired: 14 in]
      }
      frame "---------- UI ----------" {
        # "Do not put any code in this frame.\n(It is a separator no-op. You can make a copy of this frame to create a new UI frame)"
        n187 = call <vilib>:"Add State(s) to Queue__JKI_lib_State_Machine.vi"("State(s) in (\"\")"=w461) -> ("States Out"=w460:string)  [unwired: 14 in]
      }
      frame "UI: Initialize" {
        w462 = T7."Disabled and Grayed Out" ("Disabled")
        # "Disable all button on startup"
        # "Initialize the User Interface, here.\n(this is called automatically, by the Macro: Init)"
        n188 = property on="StopButton" class="Bool (strict)"("DisabledEnum"=w462) -> ()  [unwired: 2 in, 2 out]
        n189 = property on="StartButton" class="Bool (strict)"("DisabledEnum"=w462) -> ()  [unwired: 2 in, 2 out]
        n190 = property on="Video Source" class="RadioBtnsControl (strict)"("DisabledEnum"=w462) -> ()  [unwired: 2 in, 2 out]
      }
      frame "UI: showDisclaimer" {
        # "Show disclamer window.\n(It is a separator no-op. You can make a copy of this frame to create a new UI frame)"
        n191 = call <vilib>:"Application Directory.vi"() -> ("Application Directory"=w478:path)
        n192 = Build Path(base path=w478, name or relative path="Disclamer.png") -> (appended path=w476:path)
        n193 = property on="Disclamer" class="Pict"() -> ("Draw Area Size"=w474:T17)  [unwired: 2 in, 2 out]
        n194 = disable-structure "Diagram Disable Structure" shown="Disabled" {
          frame Disabled {
            n195 = flat-sequence {
              frame #0 {
                n196 = call "disclaimer.vi"() -> ()  [unwired: 12 in]
              }
              frame #1 {
                n197 = Wait (ms)(milliseconds to wait=u32 250) -> ()  [unwired: 1 out]
              }
              frame #2 {
                n198 = call "SoftwareNote.vi"() -> ()  [unwired: 12 in]
              }
            }
          }
          frame Enabled {
          }
        }
        n199 = call <vilib>:"Read PNG File.vi"("path to PNG file"=w476) -> ("image data"=w473:T18)  [unwired: 8 in, 2 out]
        n200 = Unbundle By Name(w473) -> ("Rectangle.right"=w471:i16, "Rectangle.bottom"=w469:i16)
        n201 = Unbundle By Name(w474) -> ("Width"=w472:u32, "Height"=w470:u32)
        n202 = call <vilib>:"Draw Flattened Pixmap.vi"("image data"=w473) -> ("new picture"=→"Disclamer":picture)  [unwired: 8 in]
        n203 = Divide(x=w472, y=w471) -> (x/y=w468:dbl)
        n204 = Divide(x=w470, y=w469) -> (x/y=w467:dbl)
        n205 = Max & Min(x=w468, y=w467) -> (min(x,y)=w466:dbl)  [unwired: 1 out]
        n206 = property on="Disclamer" class="Pict"("ZoomFactor"=w466) -> ()  [unwired: 2 in, 2 out]
        n207 = call <vilib>:"Add State(s) to Queue__JKI_lib_State_Machine.vi"("State(s) in (\"\")"=w482) -> ("States Out"=w481:string)  [unwired: 14 in]
      }
      frame "UI: ReadyForAquisition" {
        w487 = T7."Enabled" ("Disabled")
        # "Do not put any code in this frame.\n(It is a separator no-op. You can make a copy of this frame to create a new UI frame)"
        n208 = Unbundle By Name(w486) -> ("System Status.TCP/IP"=w485:bool, "bothVidSourceAvail"=w484:bool)
        n209 = property on="Quit" class="Bool"("DisabledEnum"=w487) -> ()  [unwired: 2 in, 2 out]
        n210 = case shown="True" w484 {
          tunnel: w487 -> [_ w492]
          frame False {
          }
          frame True {
            n211 = property on="Video Source" class="RadioBtnsControl (strict)"("DisabledEnum"=w492) -> ()  [unwired: 2 in, 2 out]
          }
        }
        n212 = property on="StartButton" class="Bool (strict)"("DisabledEnum"=w487) -> ()  [unwired: 2 in, 2 out]
        n213 = case shown="True" w485 {
          tunnel: w487 -> [_ w493]
          frame False {
          }
          frame True {
            n214 = property on="Video Display" class="Bool (strict)"("DisabledEnum"=w493) -> ()  [unwired: 2 in, 2 out]
          }
        }
        n215 = call <vilib>:"Add State(s) to Queue__JKI_lib_State_Machine.vi"("State(s) in (\"\")"=w491) -> ("States Out"=w490:string)  [unwired: 14 in]
        n216 = property on="StopButton" class="Bool (strict)"("DisabledEnum"=T7."Disabled and Grayed Out" ("Disabled")) -> ()  [unwired: 2 in, 2 out]
      }
      frame "UI: DuringAquisition" {
        w497 = T7."Disabled and Grayed Out" ("Disabled")
        # "Do not put any code in this frame.\n(It is a separator no-op. You can make a copy of this frame to create a new UI frame)"
        n217 = Unbundle By Name(w496) -> ("System Status.TCP/IP"=w495:bool, "bothVidSourceAvail"=w494:bool)
        n218 = property on="StartButton" class="Bool (strict)"("DisabledEnum"=w497) -> ()  [unwired: 2 in, 2 out]
        n219 = property on="Quit" class="Bool"("DisabledEnum"=w497) -> ()  [unwired: 2 in, 2 out]
        n220 = case shown="True" w494 {
          tunnel: w497 -> [_ w502]
          frame False {
          }
          frame True {
            n221 = property on="Video Source" class="RadioBtnsControl (strict)"("DisabledEnum"=w502) -> ()  [unwired: 2 in, 2 out]
          }
        }
        n222 = case shown="True" w495 {
          tunnel: w497 -> [_ w503]
          frame False {
          }
          frame True {
            n223 = property on="Video Display" class="Bool (strict)"("DisabledEnum"=w503) -> ()  [unwired: 2 in, 2 out]
          }
        }
        n224 = property on="StopButton" class="Bool (strict)"("DisabledEnum"=T7."Enabled" ("Disabled")) -> ()  [unwired: 2 in, 2 out]
        n225 = call <vilib>:"Add State(s) to Queue__JKI_lib_State_Machine.vi"("State(s) in (\"\")"=w501) -> ("States Out"=w500:string)  [unwired: 14 in]
      }
      frame "UI: Update" {
        # "Do not put any code in this frame.\n(It is a separator no-op. You can make a copy of this frame to create a new UI frame)"
        n226 = Unbundle By Name(w512) -> ("System Status"=→"System Hardware Connection Status":T3, "IDs.RunID"=→"Run":i8, "CaseID"=→"Case #":string, "FLImDAQ"=→"FLImDAQ":T14, "SysRunning?"=→"Aquisition Status:":bool, "IDs.BG ID"=→"BG #":i8, "IDs.Cali ID"=→"Calibration #":i8, "video source"=→"Visualization PC video source":T2)
        n227 = call <vilib>:"Add State(s) to Queue__JKI_lib_State_Machine.vi"("State(s) in (\"\")"=w515) -> ("States Out"=w514:string)  [unwired: 14 in]
      }
      frame "UI: Cursor Set" {
        # "Argument"
        # "Set and Unset Cursor Busy.\n(Usage: \"UI: Cursor Set >> Busy|Idle\")"
        n228 = case shown="\"Idle\", Default" w516 {
          tunnel: w518 -> [w523 w525]
          tunnel: [w522 w524] -> w517
          frame "Idle", Default {
            n229 = call <vilib>:"Unset Busy.vi"("error in (no error)"=w523) -> ("error out"=w522:errorcluster)  [unwired: 10 in]
          }
          frame "Busy" {
            n230 = call <vilib>:"Set Busy.vi"("error in (no error)"=w525) -> ("error out"=w524:errorcluster)  [unwired: 9 in, 1 out]
          }
        }
        n231 = call <vilib>:"Add State(s) to Queue__JKI_lib_State_Machine.vi"("State(s) in (\"\")"=w521) -> ("States Out"=w520:string)  [unwired: 14 in]
      }
      frame "UI: Front Panel State" {
        # "Argument"
        # "Set Front Panel Open or Closed\n(Usage: \"UI: Front Panel State >> Open|Close\")"
        n232 = Unbundle By Name(w528) -> ("Core.Current VI Reference"=w527:refnum<vi>)
        n233 = case shown="\"Open\", \"Standard\", Default" w526 {
          tunnel: w530 -> [w538 w553 w564 w577 w590]
          tunnel: [w540 w554 w566 w579 w592] -> w529
          tunnel: w527 -> [w539 w551 w565 w578 w591]
          frame "Open", "Standard", Default {
            w533 = T9."Standard" ("State")
            n234 = property on="Property Node" class="VI"(reference=w539, error in=w538) -> (reference out=w536:refnum<vi>, error out=w537:errorcluster, "FP.State"=w535:T9)
            n235 = Not Equal?(x=w535, y=w533) -> (x != y?=w534:bool)
            n236 = case shown="True" w534 {
              tunnel: [w544 w546] -> w540
              tunnel: w537 -> [w543 w546]
              tunnel: w536 -> [w542 _]
              tunnel: w533 -> [w541 _]
              frame True {
                n237 = invoke on="Invoke Node" class="VI" method="FP.Open"(reference=w542, error in=w543, "Activate"=TRUE, "State"=w541) -> (error out=w544:errorcluster)  [unwired: 1 in, 4 out]
              }
              frame False {
              }
            }
          }
          frame "Close", "Closed" {
            n238 = property on="Property Node" class="VI"(reference=w551, error in=w553) -> (reference out=w550:refnum<vi>, error out=w552:errorcluster, "FP.State"=w548:T9)
            n239 = Not Equal?(x=w548, y=T9."Closed" ("Front Panel Window:State")) -> (x != y?=w547:bool)
            n240 = case shown="True" w547 {
              tunnel: [w555 w558] -> w554
              tunnel: w552 -> [w555 w557]
              tunnel: w550 -> [_ w556]
              frame False {
              }
              frame True {
                n241 = invoke on="Invoke Node" class="VI" method="FP.Close"(reference=w556, error in=w557) -> (error out=w558:errorcluster)  [unwired: 1 in, 2 out]
              }
            }
          }
          frame "Hidden", "Hide" {
            w559 = T9."Hidden" ("State")
            n242 = property on="Property Node" class="VI"(reference=w565, error in=w564) -> (reference out=w562:refnum<vi>, error out=w563:errorcluster, "FP.State"=w561:T9)
            n243 = Not Equal?(x=w561, y=w559) -> (x != y?=w560:bool)
            n244 = case shown="True" w560 {
              tunnel: [w570 w571] -> w566
              tunnel: w563 -> [w569 w571]
              tunnel: w562 -> [w568 _]
              tunnel: w559 -> [w567 _]
              frame True {
                n245 = invoke on="Invoke Node" class="VI" method="FP.Open"(reference=w568, error in=w569, "State"=w567) -> (error out=w570:errorcluster)  [unwired: 2 in, 4 out]
              }
              frame False {
              }
            }
          }
          frame "Minimize", "Minimized" {
            w572 = T9."Minimized" ("State")
            n246 = property on="Property Node" class="VI"(reference=w578, error in=w577) -> (reference out=w575:refnum<vi>, error out=w576:errorcluster, "FP.State"=w574:T9)
            n247 = Not Equal?(x=w574, y=w572) -> (x != y?=w573:bool)
            n248 = case shown="True" w573 {
              tunnel: [w583 w584] -> w579
              tunnel: w576 -> [w582 w584]
              tunnel: w575 -> [w581 _]
              tunnel: w572 -> [w580 _]
              frame True {
                n249 = invoke on="Invoke Node" class="VI" method="FP.Open"(reference=w581, error in=w582, "State"=w580) -> (error out=w583:errorcluster)  [unwired: 2 in, 4 out]
              }
              frame False {
              }
            }
          }
          frame "Maximize", "Maximized" {
            w585 = T9."Maximized" ("State")
            n250 = property on="Property Node" class="VI"(reference=w591, error in=w590) -> (reference out=w588:refnum<vi>, error out=w589:errorcluster, "FP.State"=w587:T9)
            n251 = Not Equal?(x=w587, y=w585) -> (x != y?=w586:bool)
            n252 = case shown="True" w586 {
              tunnel: [w596 w597] -> w592
              tunnel: w589 -> [w595 w597]
              tunnel: w588 -> [w594 _]
              tunnel: w585 -> [w593 _]
              frame True {
                n253 = invoke on="Invoke Node" class="VI" method="FP.Open"(reference=w594, error in=w595, "State"=w593) -> (error out=w596:errorcluster)  [unwired: 2 in, 4 out]
              }
              frame False {
              }
            }
          }
        }
        n254 = call <vilib>:"Add State(s) to Queue__JKI_lib_State_Machine.vi"("State(s) in (\"\")"=w532) -> ("States Out"=w531:string)  [unwired: 14 in]
      }
      frame "---------- Utility ----------" {
        # "Template Separator\n(You can make a copy of, or modify, this frame)"
        n255 = call <vilib>:"Add State(s) to Queue__JKI_lib_State_Machine.vi"("State(s) in (\"\")"=w601) -> ("States Out"=w600:string)  [unwired: 14 in]
      }
      frame "Utility: StartBeep" {
        # "Beep\n([Covers: REQ18])"
        n256 = call <vilib>:"Beep.vi"("use system alert? (T)"=FALSE, "duration (msec)"=u32 1000, "frequency (Hz)"=u32 2000) -> ()  [unwired: 9 in]
        n257 = call <vilib>:"Add State(s) to Queue__JKI_lib_State_Machine.vi"("State(s) in (\"\")"=w608) -> ("States Out"=w607:string)  [unwired: 14 in]
      }
      frame "Utility: EndBeep" {
        # "Beep\n([Covers: REQ18])"
        n258 = flat-sequence {
          frame #0 {
            n259 = call <vilib>:"Beep.vi"("use system alert? (T)"=FALSE, "duration (msec)"=u32 500, "frequency (Hz)"=u32 2000) -> ()  [unwired: 9 in]
          }
          frame #1 {
            n260 = call <vilib>:"Beep.vi"("use system alert? (T)"=FALSE, "duration (msec)"=u32 500, "frequency (Hz)"=u32 2000) -> ()  [unwired: 9 in]
          }
        }
        n261 = call <vilib>:"Add State(s) to Queue__JKI_lib_State_Machine.vi"("State(s) in (\"\")"=w612) -> ("States Out"=w611:string)  [unwired: 14 in]
      }
      frame "Utility: Dewelling" {
        # "Main loop dewell\n(Dewelling >> #)"
        n262 = Fract/Exp String To Number(string=w622, default (0 dbl)=0) -> (number=w620:i32)  [unwired: 2 in, 1 out]
        n263 = Wait (ms)(milliseconds to wait=w620) -> ()  [unwired: 1 out]
        n264 = call <vilib>:"Add State(s) to Queue__JKI_lib_State_Machine.vi"("State(s) in (\"\")"=w625) -> ("States Out"=w624:string)  [unwired: 14 in]
      }
      frame "---------- SysLog ----------" {
        # "Template Separator\n(You can make a copy of, or modify, this frame)"
        n265 = call <vilib>:"Add State(s) to Queue__JKI_lib_State_Machine.vi"("State(s) in (\"\")"=w629) -> ("States Out"=w628:string)  [unwired: 14 in]
      }
      frame "SysLog: OpenLogFile" {
        # "Template Separator\n(You can make a copy of, or modify, this frame)"
        n266 = call <vilib>:"Add State(s) to Queue__JKI_lib_State_Machine.vi"("State(s) in (\"\")"=w633) -> ("States Out"=w632:string)  [unwired: 14 in]
      }
      frame "---------- TCP ----------" {
        # "Template Separator\n(You can make a copy of, or modify, this frame)"
        n267 = call <vilib>:"Add State(s) to Queue__JKI_lib_State_Machine.vi"("State(s) in (\"\")"=w637) -> ("States Out"=w636:string)  [unwired: 14 in]
      }
      frame "TCP: Initialize" {
        # "Initialize TCP connection to aimging beam computer\n(You can make a copy of, or modify, this frame)"
        n268 = call <vilib>:"TCP Listen.vi"("resolve remote address (T)"=TRUE, "error in (no error)"=w662, "timeout ms (wait forever: -1)"=500, "port"=u16 2100, "service name"="RTLT") -> ("error out"=w657:errorcluster, "remote address"=→"remote address":string, "connection ID"=w658:refnum<k5>, "listener ID"=w642:refnum<k5>)  [unwired: 2 in, 1 out]
        n269 = TCP Read(connection ID=w658, bytes to read=512, error in (no error)=w657, 7:T11."CRLF" ("mode (standard)"), 9:5000 ("timeout ms (25000)")) -> (connection ID out=w648:refnum<k5>, data out=w654:string, error out=w649:errorcluster)
        n270 = Concatenate Strings("alive" ("string"), "\r\n" ("End of Line Constant")) -> (w652:string)
        n271 = Equal?(x=w654, y=w652) -> (x = y?=w650:bool)
        n272 = case shown="True" w650 {
          tunnel: w649 -> [w666 w687]
          tunnel: w648 -> [_ w681]
          tunnel: [w667 w685] -> w647
          tunnel: w645 -> [w673 _]
          tunnel: [w669 0] -> w644
          tunnel: [w668 "" ("Empty String Constant")] -> w643
          tunnel: [FALSE TRUE] -> w638
          frame False {
            # "if unsuccessful and count <10, increament count \nand try again"
            n273 = Unbundle By Name(w673) -> ("TCP attempt count"=w670:i32)
            n274 = Less?(x=w670, y=6) -> (x < y?=w671:bool)
            n275 = case shown="True" w671 {
              tunnel: w670 -> [w676 w680]
              tunnel: [w676 w679] -> w669
              tunnel: ["" ("Empty String Constant") "TCP: Initialize"] -> w668
              tunnel: [errorcluster {"status"=TRUE, "code"=5001, "source"="TCP/IP"} ("error in (no error)") errorcluster {"status"=FALSE, "code"=5001, "source"=""} ("error in (no error)")] -> w667
              tunnel: w666 -> [_ _]
              frame False {
                # "send error and shut down"
              }
              frame True {
                # "try again until 10th"
                n276 = Increment(x=w680) -> (x+1=w679:i32)
              }
            }
          }
          frame True {
            # "if connection is successful\nwrite TCP FVG"
            n277 = call "TcpIDFGV.vi"("Error In"=w687, "action"=enum16{"write", "read"}."write", "connection ID in"=w681) -> ("Error Out"=w685:errorcluster)  [unwired: 7 in, 1 out]
          }
        }
        n278 = global write "GlobalVariables.vi" "TCP connected?"(w638) -> ()
        n279 = Bundle By Name(cluster=w645, "TCP attempt count"=w644, "System Status.TCP/IP"=w638, "listener ID"=w642) -> (w646:T12)
        n280 = call <vilib>:"Add State(s) to Queue__JKI_lib_State_Machine.vi"("State(s) in Front (\"\")"=w643, "State(s) in (\"\")"=w664) -> ("States Out"=w663:string)  [unwired: 13 in]
      }
      frame "TCP: InitNew" {
        # "if unsuccessful and count <10, increament count \nand try again"
        # "Initialize TCP connection to aimging beam computer\n(You can make a copy of, or modify, this frame)"
        n281 = TCP Create Listener(10:u16 2100 ("port"), 11:"RTLT" ("service name")) -> (0:w696:errorcluster, 3:w688:refnum<k5>)  [unwired: 3 in, 1 out]
        n282 = while {
          tunnel: w688 -> [w715]
          tunnel: w696 -> [w714]
          tunnel: [w705] -> w694
          tunnel: [w702] -> w690
          i -> [w711]
          stop <- w702 stop-if-true
          n283 = TCP Wait On Listener(8:w714, 9:100 ("timeout ms (wait forever: -1)"), 11:w715) -> (0:w712:errorcluster, 4:w709:refnum<k5>)  [unwired: 1 in, 3 out]
          n284 = Less Or Equal?(x=100, y=w711) -> (x <= y?=w708:bool)
          n285 = case shown="No Error" w712 {
            selector: w712 -> [w725 w735]
            tunnel: w709 -> [w726 _]
            tunnel: [errorcluster {"status"=TRUE, "code"=0, "source"=""} ("No error") w736] -> w704
            tunnel: [w717 FALSE ("TCP connected?")] -> w705
            frame No Error {
              # "connection is ready, read data"
              n286 = TCP Read(connection ID=w726, bytes to read=512, error in (no error)=w725, 7:T11."CRLF" ("mode (standard)"), 9:5000 ("timeout ms (25000)")) -> (connection ID out=w719:refnum<k5>, data out=w721:string, error out=w718:errorcluster)
              n287 = Concatenate Strings("alive" ("string"), "\r\n" ("End of Line Constant")) -> (w722:string)
              n288 = Equal?(x=w722, y=w721) -> (x = y?=w720:bool)
              n289 = case shown="False" w720 {
                tunnel: w719 -> [_ w731]
                tunnel: w718 -> [_ _]
                tunnel: [FALSE ("TCP connected?") TRUE ("TCP connected?")] -> w717
                frame False {
                }
                frame True {
                  n290 = call "TcpIDFGV.vi"("action"=enum16{"write", "read"}."write", "connection ID in"=w731) -> ()  [unwired: 8 in, 2 out]
                }
              }
            }
            frame Error {
              # "connection not ready, keep waiting"
              n291 = Unbundle By Name(w735) -> ("code"=w737:i32)
              n292 = case shown="56" w737 {
                tunnel: w735 -> [w738 _]
                tunnel: [w738 w739] -> w736
                frame Default {
                }
                frame 56 {
                  w739 = errorcluster {"status"=FALSE, "code"=0, "source"=""}  # No error
                }
              }
            }
          }
          n293 = Select(t=errorcluster {"status"=TRUE, "code"=5001, "source"=""} ("error in (no error)"), s=w708, f=errorcluster {"status"=FALSE, "code"=0, "source"=""} ("error in (no error)")) -> (s? t:f=w703:errorcluster)
          n294 = Merge Errors(w704, w703) -> (w702:errorcluster)
        }
        n295 = Unbundle By Name(w690) -> ("code"=w693:i32)
        n296 = Bundle By Name(cluster=w695, "System Status.TCP/IP"=w694, "listener ID"=w688) -> (w699:T12)
        n297 = global write "GlobalVariables.vi" "TCP connected?"(w694) -> ()
        n298 = Equal To 0?(x=w693) -> (x = 0?=w692:bool)
        n299 = Select(t=errorcluster {"status"=FALSE, "code"=0, "source"=""} ("error in (no error)"), s=w692, f=w690) -> (s? t:f=w689:errorcluster)
        n300 = call <vilib>:"Add State(s) to Queue__JKI_lib_State_Machine.vi"("State(s) in (\"\")"=w701) -> ("States Out"=w700:string)  [unwired: 14 in]
      }
      frame "TCP: checkSource" {
        # "Check visualization PC video source\n(send !video_source message, listen for response, then parse it to binary mask)"
        n301 = Unbundle By Name(w746) -> ("System Status.TCP/IP"=w749:bool)
        n302 = case shown="True" w749 {
          tunnel: w748 -> [w753 w776]
          tunnel: [w753 w760] -> w747
          tunnel: [w752 w765] -> w744
          tunnel: [w752 w763] -> w743
          tunnel: [w752 w764] -> w742
          tunnel: [w752 w762] -> w741
          tunnel: [w752 w754] -> w740
          frame False {
            w752 = FALSE
          }
          frame True {
            n303 = call "TcpIDFGV.vi"("Error In"=w776, "action"=enum16{"write", "read"}."read") -> ("Error Out"=w773:errorcluster, "connection ID out"=w775:refnum<k5>)  [unwired: 8 in]
            n304 = call "TCP_WriteRead.vi"("error in (no error)"=w773, "data in"="!video_source", "connectin ID in"=w775) -> ("error out"=w770:errorcluster, "data out"=w772:string)  [unwired: 4 in, 1 out]
            n305 = Scan From String(format string="!video_source:%d", input string=w772, error in=w770) -> (error out=w761:errorcluster, output 1=w759:i32)  [unwired: 2 in, 2 out]
            n306 = case shown="5..7, 9..11, 13..15" w759 {
              tunnel: w761 -> [_ _ _ _]
              tunnel: [errorcluster {"status"=TRUE, "code"=5007, "source"="Visualization PC"} ("error out") errorcluster {"status"=FALSE, "code"=0, "source"=""} ("error out") errorcluster {"status"=FALSE, "code"=0, "source"=""} ("error out") errorcluster {"status"=FALSE, "code"=0, "source"=""} ("error out")] -> w760
              tunnel: [FALSE FALSE FALSE TRUE] -> w754
              frame 0, Default {
                # "No video source available or default"
                n307 = property on="Video Source" class="RadioBtnsControl (strict)"("DisabledEnum"=T7."Disabled and Grayed Out" ("Disabled")) -> ()  [unwired: 2 in, 2 out]
              }
              frame 1..3 {
                # "one or both camera available"
                n308 = local write "Video Source"(enum32{"Camera", "FrameGrabber"}."Camera" ("Video Source")) -> ()
                n309 = property on="Video Source" class="RadioBtnsControl (strict)"("DisabledEnum"=T7."Disabled and Grayed Out" ("Disabled")) -> ()  [unwired: 2 in, 2 out]
              }
              frame 4, 8, 12 {
                # "one or both frame grabber available"
                n310 = local write "Video Source"(enum32{"Camera", "FrameGrabber"}."FrameGrabber" ("Video Source")) -> ()
                n311 = property on="Video Source" class="RadioBtnsControl (strict)"("DisabledEnum"=T7."Disabled and Grayed Out" ("Disabled")) -> ()  [unwired: 2 in, 2 out]
              }
              frame 5..7, 9..11, 13..15 {
                n312 = property on="Video Source" class="RadioBtnsControl (strict)"("DisabledEnum"=T7."Enabled" ("Disabled")) -> ()  [unwired: 2 in, 2 out]
              }
            }
            n313 = Integer to Fixed-Point Cast(fixed-point type=fxp<+,4,4> 0.0, integer=w759) -> (fixed-point=w758:fxp<+,4,4>)
            n314 = Number To Boolean Array(number=w758) -> (Boolean array=w756:bool[])
            n315 = Reverse 1D Array(array=w756) -> (reversed array=w755:bool[])
            n316 = Index Array(array=w755, index=0) -> (element=w765:bool)
            n317 = Index Array(array=w755, index=1) -> (element=w763:bool)
            n318 = Index Array(array=w755, index=2) -> (element=w764:bool)
            n319 = Index Array(array=w755, index=3) -> (element=w762:bool)
          }
        }
        n320 = Bundle By Name(cluster=w746, "video source.Main Frame Grabber"=w744, "video source.Side Frame Grabber"=w743, "video source.Main Camera"=w742, "video source.Side Camera"=w741, "bothVidSourceAvail"=w740) -> (w745:T12)
        n321 = call <vilib>:"Add State(s) to Queue__JKI_lib_State_Machine.vi"("State(s) in (\"\")"=w751) -> ("States Out"=w750:string)  [unwired: 14 in]
      }
      frame "TCP: SyncTime" {
        # "Template Separator\n(You can make a copy of, or modify, this frame)"
        n322 = Unbundle By Name(w793) -> ("System Status.TCP/IP"=w792:bool)
        n323 = case shown="True" w792 {
          tunnel: w794 -> [_ w801]
          frame False {
          }
          frame True {
            n324 = call "TcpIDFGV.vi"("Error In"=w801, "action"=enum16{"write", "read"}."read") -> ("Error Out"=w800:errorcluster, "connection ID out"=w797:refnum<k5>)  [unwired: 8 in]
            n325 = call <userlib>:"Tick Count (ms)__ogtk.vi"("error in (no error)"=w800) -> ("error out"=w799:errorcluster, "millisecond timer value"=w798:u32)  [unwired: 9 in]
            n326 = while {
              tunnel: w799 -> [w821]
              tunnel: w797 -> [w820]
              tunnel: w798 -> [w809]
              stop <- w804 stop-if-true
              n327 = Concatenate Strings("latencycheck" ("string"), "\r\n" ("End of Line Constant")) -> (w816:string)
              n328 = TCP Read(connection ID=w820, bytes to read=512, error in (no error)=w821, 7:T11."CRLF" ("mode (standard)"), 9:2000 ("timeout ms (25000)")) -> (connection ID out=w813:refnum<k5>, data out=w811:string, error out=w803:errorcluster)
              n329 = Tick Count (ms)() -> (millisecond timer value=w810:u32)
              n330 = Subtract(x=w810, y=w809) -> (x-y=w808:u32)
              n331 = Equal?(x=w811, y=w816) -> (x = y?=w812:bool)
              n332 = case shown="False" w812 {
                tunnel: w813 -> [_ w834]
                tunnel: w811 -> [w826 _]
                tunnel: [w822 FALSE] -> w806
                tunnel: w803 -> [_ w828]
                frame False {
                  n333 = Concatenate Strings("synctimer" ("string"), "\r\n" ("End of Line Constant")) -> (w823:string)
                  n334 = Equal?(x=w826, y=w823) -> (x = y?=w822:bool)
                  "Sync Success?" <- w822
                }
                frame True {
                  n335 = Concatenate Strings("latencycheck:" ("string"), "\r\n" ("End of Line Constant")) -> (w833:string)
                  n336 = TCP Write(connection ID=w834, data in=w833, error in (no error)=w828, 9:1000 ("timeout ms (25000)")) -> (error out=w827:errorcluster)  [unwired: 2 out]
                  n337 = call <vilib>:"Clear Errors.vi"("error in (no error)"=w827) -> ()  [unwired: 5 in, 2 out]
                }
              }
              n338 = Greater?(x=w808, y=u32 10000 ("x-y")) -> (0:w805:bool)
              n339 = Or(x=w806, y=w805) -> (x .or. y?=w804:bool)
            }
          }
        }
        n340 = call <vilib>:"Add State(s) to Queue__JKI_lib_State_Machine.vi"("State(s) in (\"\")"=w796) -> ("States Out"=w795:string)  [unwired: 14 in]
      }
      frame "TCP: SendSettingMacro" {
        # "Template Separator\n(You can make a copy of, or modify, this frame)"
        n341 = Unbundle By Name(w837) -> ("System Status.TCP/IP"=w836:bool)
        n342 = case shown="True" w836 {
          tunnel: ["" ("Empty String Constant") "TCP: sendSubjectID\nTCP: sendScaleBarSetting\nTCP: sendScaleMaxMin\nTCP: sendDeconChannel\nTCP: sendANSI\nTCP: sendRadius\nTCP: send3Dsetting\nTCP: sendFirefly\nTCP: sendPentero"] -> w835
          frame False {
          }
          frame True {
          }
        }
        n343 = call <vilib>:"Add State(s) to Queue__JKI_lib_State_Machine.vi"("State(s) in Front (\"\")"=w835, "State(s) in (\"\")"=w840) -> ("States Out"=w839:string)  [unwired: 13 in]
      }
      frame "TCP: sendRunNum" {
        # "Send run number to AB PC\n(You can make a copy of, or modify, this frame)"
        n344 = Unbundle By Name(w847) -> ("System Status.TCP/IP"=w844:bool, "IDs.RunID"=w848:i8)
        n345 = Increment(x=w848) -> (x+1=w843:i8)
        n346 = case shown="True" w844 {
          tunnel: w843 -> [_ w861]
          tunnel: [w851 w853] -> w846
          tunnel: w845 -> [w851 w852]
          frame False {
          }
          frame True {
            n347 = Number To Decimal String(number=w861, width (-)=i16 3) -> (decimal integer string=w856:string)
            n348 = call "TcpIDFGV.vi"("Error In"=w852, "action"=enum16{"write", "read"}."read") -> ("Error Out"=w854:errorcluster, "connection ID out"=w858:refnum<k5>)  [unwired: 8 in]
            n349 = Concatenate Strings("!run:", w856) -> (w855:string)
            n350 = call "TCP_WriteRead.vi"("error in (no error)"=w854, "data in"=w855, "connectin ID in"=w858) -> ("error out"=w853:errorcluster)  [unwired: 4 in, 2 out]
          }
        }
        n351 = call <vilib>:"Add State(s) to Queue__JKI_lib_State_Machine.vi"("State(s) in (\"\")"=w850) -> ("States Out"=w849:string)  [unwired: 14 in]
      }
      frame "TCP: sendVideoSource" {
        # "Send video source \n(You can make a copy of, or modify, this frame)"
        n352 = Unbundle By Name(w863) -> ("System Status.TCP/IP"=w862:bool)
        n353 = case shown="True" w862 {
          tunnel: [w868 w870] -> w865
          tunnel: w864 -> [w868 w869]
          frame False {
          }
          frame True {
            n354 = case shown="\"Camera\", Default" "Video Source" {
              tunnel: [0 1] -> w875
              frame "Camera", Default {
              }
              frame "FrameGrabber" {
              }
            }
            n355 = call "TcpIDFGV.vi"("Error In"=w869, "action"=enum16{"write", "read"}."read") -> ("Error Out"=w871:errorcluster, "connection ID out"=w877:refnum<k5>)  [unwired: 8 in]
            n356 = Number To Decimal String(number=w875) -> (decimal integer string=w873:string)  [unwired: 1 in]
            n357 = Concatenate Strings("!invivo:" ("data in"), w873) -> (w872:string)
            n358 = call "TCP_WriteRead.vi"("error in (no error)"=w871, "data in"=w872, "connectin ID in"=w877) -> ("error out"=w870:errorcluster)  [unwired: 4 in, 2 out]
          }
        }
        n359 = call <vilib>:"Add State(s) to Queue__JKI_lib_State_Machine.vi"("State(s) in (\"\")"=w867) -> ("States Out"=w866:string)  [unwired: 14 in]
      }
      frame "TCP: startRun" {
        # "Template Separator\n(You can make a copy of, or modify, this frame)"
        n360 = Unbundle By Name(w882) -> ("System Status.TCP/IP"=w881:bool)
        n361 = case shown="True" w881 {
          tunnel: [w887 w889] -> w884
          tunnel: w883 -> [w887 w888]
          frame False {
          }
          frame True {
            n362 = call "TcpIDFGV.vi"("Error In"=w888, "action"=enum16{"write", "read"}."read") -> ("Error Out"=w890:errorcluster, "connection ID out"=w891:refnum<k5>)  [unwired: 8 in]
            n363 = call "TCP_WriteRead.vi"("error in (no error)"=w890, "data in"="!acquire:1", "connectin ID in"=w891) -> ("error out"=w889:errorcluster)  [unwired: 4 in, 2 out]
          }
        }
        n364 = call <vilib>:"Add State(s) to Queue__JKI_lib_State_Machine.vi"("State(s) in (\"\")"=w886) -> ("States Out"=w885:string)  [unwired: 14 in]
      }
      frame "TCP: stopRun" {
        # "Send stop run to AB PC\n(You can make a copy of, or modify, this frame)"
        n365 = Unbundle By Name(w895) -> ("System Status.TCP/IP"=w894:bool)
        n366 = case shown="True" w894 {
          tunnel: [w900 w902] -> w897
          tunnel: w896 -> [w900 w901]
          frame False {
            # "if not connected, do nothing"
          }
          frame True {
            # "If TCP connected, send stop run"
            n367 = call "TcpIDFGV.vi"("Error In"=w901, "action"=enum16{"write", "read"}."read") -> ("Error Out"=w903:errorcluster, "connection ID out"=w905:refnum<k5>)  [unwired: 8 in]
            n368 = call "TCP_WriteRead.vi"("error in (no error)"=w903, "data in"="!acquire:0", "connectin ID in"=w905) -> ("error out"=w902:errorcluster)  [unwired: 4 in, 2 out]
          }
        }
        n369 = call <vilib>:"Add State(s) to Queue__JKI_lib_State_Machine.vi"("State(s) in (\"\")"=w899) -> ("States Out"=w898:string)  [unwired: 14 in]
      }
      frame "TCP: SyncTimer" {
        # "Template Separator\n(You can make a copy of, or modify, this frame)"
        n370 = call "TcpIDFGV.vi"("Error In"=w912, "action"=enum16{"write", "read"}."read") -> ("Error Out"=w913:errorcluster, "connection ID out"=w914:refnum<k5>)  [unwired: 8 in]
        n371 = while {
          tunnel: w914 -> [w932]
          shift-right: [w927] -> w908
          shift-left: w913 -> [w928]
          tunnel: [w919] -> w911
          i -> [w924]
          stop <- w922 stop-if-true
          n372 = TCP Read(connection ID=w932, bytes to read=512, error in (no error)=w928, 7:T11."CRLF" ("mode (standard)"), 9:1000 ("timeout ms (25000)")) -> (connection ID out=w919:refnum<k5>, data out=w926:string, error out=w927:errorcluster)
          "syctimer data out" <- w926
          n373 = Equal?(x="!synctimer:", y=w926) -> (x = y?=w921:bool)
          n374 = Greater?(x=w924, y=10000) -> (0:w920:bool)
          n375 = Or(x=w921, y=w920) -> (x .or. y?=w922:bool)
        }
        n376 = TCP Write(connection ID=w911, data in="!synctimer:", error in (no error)=w908, 9:1000 ("timeout ms (25000)")) -> (error out=w907:errorcluster)  [unwired: 2 out]
        n377 = call <vilib>:"Add State(s) to Queue__JKI_lib_State_Machine.vi"("State(s) in (\"\")"=w918) -> ("States Out"=w917:string)  [unwired: 14 in]
      }
      frame "TCP: sendSubjectID" {
        # "Send subject ID"
        n378 = Unbundle By Name(w934) -> ("System Status.TCP/IP"=w933:bool, "CaseID"=w937:string)
        n379 = case shown="True" w933 {
          tunnel: w937 -> [_ w947]
          tunnel: [w940 w942] -> w936
          tunnel: w935 -> [w940 w941]
          frame False {
          }
          frame True {
            n380 = call "TcpIDFGV.vi"("Error In"=w941, "action"=enum16{"write", "read"}."read") -> ("Error Out"=w943:errorcluster, "connection ID out"=w945:refnum<k5>)  [unwired: 8 in]
            n381 = Concatenate Strings("!subject:", w947) -> (w944:string)
            n382 = call "TCP_WriteRead.vi"("error in (no error)"=w943, "data in"=w944, "connectin ID in"=w945) -> ("error out"=w942:errorcluster)  [unwired: 4 in, 2 out]
          }
        }
        n383 = call <vilib>:"Add State(s) to Queue__JKI_lib_State_Machine.vi"("State(s) in (\"\")"=w939) -> ("States Out"=w938:string)  [unwired: 14 in]
      }
      frame "TCP: sendScaleBarSetting" {
        # "Template Separator\n(You can make a copy of, or modify, this frame)"
        n384 = Unbundle By Name(w951) -> ("System Status.TCP/IP"=w949:bool, "VideoConfig.Scale Bar"=w950:bool)
        n385 = case shown="True" w949 {
          tunnel: [w956 w964] -> w953
          tunnel: w952 -> [w956 w963]
          tunnel: w950 -> [_ w962]
          frame False {
          }
          frame True {
            n386 = Boolean To (0,1)(Boolean=w962) -> (0, 1=w961:i16)
            n387 = call "TcpIDFGV.vi"("Error In"=w963, "action"=enum16{"write", "read"}."read") -> ("Error Out"=w965:errorcluster, "connection ID out"=w966:refnum<k5>)  [unwired: 8 in]
            n388 = Number To Fractional String(number=w961, width (-)=i16 1) -> (F-format string=w959:string)  [unwired: 2 in]
            n389 = Concatenate Strings("!autocolor:" ("data in"), w959) -> (w957:string)
            n390 = call "TCP_WriteRead.vi"("error in (no error)"=w965, "data in"=w957, "connectin ID in"=w966) -> ("error out"=w964:errorcluster)  [unwired: 4 in, 2 out]
          }
        }
        n391 = call <vilib>:"Add State(s) to Queue__JKI_lib_State_Machine.vi"("State(s) in (\"\")"=w955) -> ("States Out"=w954:string)  [unwired: 14 in]
      }
      frame "TCP: sendScaleMaxMin" {
        # "Send scale bar max and min to AB PC\n(You can make a copy of, or modify, this frame)"
        n392 = Unbundle By Name(w971) -> ("System Status.TCP/IP"=w968:bool, "VideoConfig.Scale Low"=w970:dbl, "VideoConfig.Scale High"=w969:dbl)
        n393 = case shown="True" w968 {
          tunnel: [w976 w989] -> w973
          tunnel: w972 -> [w976 w988]
          tunnel: w970 -> [_ w987]
          tunnel: w969 -> [_ w978]
          frame False {
          }
          frame True {
            n394 = call "TcpIDFGV.vi"("Error In"=w988, "action"=enum16{"write", "read"}."read") -> ("Error Out"=w990:errorcluster, "connection ID out"=w991:refnum<k5>)  [unwired: 8 in]
            n395 = Number To Fractional String(number=w987, width (-)=i16 4, precision (6)=i16 2) -> (F-format string=w983:string)  [unwired: 1 in]
            n396 = Number To Fractional String(number=w978, width (-)=i16 4, precision (6)=i16 2) -> (F-format string=w979:string)  [unwired: 1 in]
            n397 = Concatenate Strings("!color:" ("string"), w983, ";" ("string"), w979) -> (w977:string)
            n398 = call "TCP_WriteRead.vi"("error in (no error)"=w990, "data in"=w977, "connectin ID in"=w991) -> ("error out"=w989:errorcluster)  [unwired: 4 in, 2 out]
          }
        }
        n399 = call <vilib>:"Add State(s) to Queue__JKI_lib_State_Machine.vi"("State(s) in (\"\")"=w975) -> ("States Out"=w974:string)  [unwired: 14 in]
      }
      frame "TCP: sendDeconChannel" {
        # "Send Decon channel\n(You can make a copy of, or modify, this frame)"
        n400 = Unbundle By Name(w994) -> ("System Status.TCP/IP"=w993:bool)
        n401 = case shown="True" w993 {
          tunnel: [w999 w1004] -> w996
          tunnel: w995 -> [w999 w1003]
          frame False {
          }
          frame True {
            n402 = local read "Channel"() -> (w1002:enum16{"Ch1", "Ch2", "Ch3"})
            n403 = Increment(x=w1002) -> (x+1=w1001:enum16{"Ch1", "Ch2", "Ch3"})
            n404 = Number To Decimal String(number=w1001) -> (decimal integer string=w1000:string)  [unwired: 1 in]
            n405 = call "TcpIDFGV.vi"("Error In"=w1003, "action"=enum16{"write", "read"}."read") -> ("Error Out"=w1005:errorcluster, "connection ID out"=w1008:refnum<k5>)  [unwired: 8 in]
            n406 = Concatenate Strings("!channel:", w1000) -> (w1006:string)
            n407 = call "TCP_WriteRead.vi"("error in (no error)"=w1005, "data in"=w1006, "connectin ID in"=w1008) -> ("error out"=w1004:errorcluster)  [unwired: 4 in, 2 out]
          }
        }
        n408 = call <vilib>:"Add State(s) to Queue__JKI_lib_State_Machine.vi"("State(s) in (\"\")"=w998) -> ("States Out"=w997:string)  [unwired: 14 in]
      }
      frame "TCP: sendANSI" {
        # "Template Separator\n(You can make a copy of, or modify, this frame)"
        n409 = Unbundle By Name(w1012) -> ("System Status.TCP/IP"=w1010:bool, "VideoConfig.ANSI"=w1011:dbl)
        n410 = case shown="False" w1010 {
          tunnel: [w1017 w1023] -> w1014
          tunnel: w1013 -> [w1017 w1022]
          tunnel: w1011 -> [_ w1021]
          frame False {
          }
          frame True {
            n411 = Number To Fractional String(number=w1021) -> (F-format string=w1019:string)  [unwired: 3 in]
            n412 = call "TcpIDFGV.vi"("Error In"=w1022, "action"=enum16{"write", "read"}."read") -> ("Error Out"=w1024:errorcluster, "connection ID out"=w1025:refnum<k5>)  [unwired: 8 in]
            n413 = Concatenate Strings("!ansi:" ("data in"), w1019) -> (w1018:string)
            n414 = call "TCP_WriteRead.vi"("error in (no error)"=w1024, "data in"=w1018, "connectin ID in"=w1025) -> ("error out"=w1023:errorcluster)  [unwired: 4 in, 2 out]
          }
        }
        n415 = call <vilib>:"Add State(s) to Queue__JKI_lib_State_Machine.vi"("State(s) in (\"\")"=w1016) -> ("States Out"=w1015:string)  [unwired: 14 in]
      }
      frame "TCP: sendRadius" {
        # "Send drawing radius to AB PC\n(You can make a copy of, or modify, this frame)"
        n416 = Unbundle By Name(w1029) -> ("System Status.TCP/IP"=w1027:bool, "VideoConfig.Radius"=w1028:dbl)
        n417 = case shown="False" w1027 {
          tunnel: [w1034 w1040] -> w1031
          tunnel: w1030 -> [w1034 w1039]
          tunnel: w1028 -> [_ w1038]
          frame False {
          }
          frame True {
            n418 = Number To Fractional String(number=w1038) -> (F-format string=w1037:string)  [unwired: 3 in]
            n419 = Concatenate Strings("!radius:" ("data in"), w1037) -> (w1035:string)
            n420 = call "TcpIDFGV.vi"("Error In"=w1039, "action"=enum16{"write", "read"}."read") -> ("Error Out"=w1041:errorcluster, "connection ID out"=w1042:refnum<k5>)  [unwired: 8 in]
            n421 = call "TCP_WriteRead.vi"("error in (no error)"=w1041, "data in"=w1035, "connectin ID in"=w1042) -> ("error out"=w1040:errorcluster)  [unwired: 4 in, 2 out]
          }
        }
        n422 = call <vilib>:"Add State(s) to Queue__JKI_lib_State_Machine.vi"("State(s) in (\"\")"=w1033) -> ("States Out"=w1032:string)  [unwired: 14 in]
      }
      frame "TCP: send3Dsetting" {
        # "Send 3D setting to AB computer\n(You can make a copy of, or modify, this frame)"
        n423 = Unbundle By Name(w1046) -> ("System Status.TCP/IP"=w1044:bool, "VideoConfig.3D?"=w1045:bool)
        n424 = case shown="True" w1044 {
          tunnel: [w1051 w1058] -> w1048
          tunnel: w1047 -> [w1051 w1057]
          tunnel: w1045 -> [_ w1056]
          frame False {
          }
          frame True {
            n425 = Boolean To (0,1)(Boolean=w1056) -> (0, 1=w1055:i16)
            n426 = Number To Fractional String(number=w1055) -> (F-format string=w1054:string)  [unwired: 3 in]
            n427 = call "TcpIDFGV.vi"("Error In"=w1057, "action"=enum16{"write", "read"}."read") -> ("Error Out"=w1059:errorcluster, "connection ID out"=w1060:refnum<k5>)  [unwired: 8 in]
            n428 = Concatenate Strings("!3dset:" ("data in"), w1054) -> (w1052:string)
            n429 = call "TCP_WriteRead.vi"("error in (no error)"=w1059, "data in"=w1052, "connectin ID in"=w1060) -> ("error out"=w1058:errorcluster)  [unwired: 4 in, 2 out]
          }
        }
        n430 = call <vilib>:"Add State(s) to Queue__JKI_lib_State_Machine.vi"("State(s) in (\"\")"=w1050) -> ("States Out"=w1049:string)  [unwired: 14 in]
      }
      frame "TCP: sendFirefly" {
        # "Template Separator\n(You can make a copy of, or modify, this frame)"
        n431 = Unbundle By Name(w1063) -> ("System Status.TCP/IP"=w1062:bool)
        n432 = case shown="False" w1062 {
          tunnel: [w1068 w1070] -> w1065
          tunnel: w1064 -> [w1068 w1069]
          frame False {
          }
          frame True {
            n433 = call "TcpIDFGV.vi"("Error In"=w1069, "action"=enum16{"write", "read"}."read") -> ("Error Out"=w1071:errorcluster, "connection ID out"=w1073:refnum<k5>)  [unwired: 8 in]
            n434 = call "TCP_WriteRead.vi"("error in (no error)"=w1071, "data in"="!firefly:0", "connectin ID in"=w1073) -> ("error out"=w1070:errorcluster)  [unwired: 4 in, 2 out]
          }
        }
        n435 = call <vilib>:"Add State(s) to Queue__JKI_lib_State_Machine.vi"("State(s) in (\"\")"=w1067) -> ("States Out"=w1066:string)  [unwired: 14 in]
      }
      frame "TCP: sendPentero" {
        # "Send Pentero setting to AB computer\n(You can make a copy of, or modify, this frame)"
        n436 = Unbundle By Name(w1076) -> ("System Status.TCP/IP"=w1075:bool)
        n437 = case shown="True" w1075 {
          tunnel: [w1081 w1083] -> w1078
          tunnel: w1077 -> [w1081 w1082]
          frame False {
          }
          frame True {
            n438 = call "TcpIDFGV.vi"("Error In"=w1082, "action"=enum16{"write", "read"}."read") -> ("Error Out"=w1084:errorcluster, "connection ID out"=w1086:refnum<k5>)  [unwired: 8 in]
            n439 = call "TCP_WriteRead.vi"("error in (no error)"=w1084, "data in"="!pentero:0", "connectin ID in"=w1086) -> ("error out"=w1083:errorcluster)  [unwired: 4 in, 2 out]
          }
        }
        n440 = call <vilib>:"Add State(s) to Queue__JKI_lib_State_Machine.vi"("State(s) in (\"\")"=w1080) -> ("States Out"=w1079:string)  [unwired: 14 in]
      }
      frame "TCP: sendChannel" {
        # "Send DeCon Channel to AB computer\n()"
        n441 = Unbundle By Name(w1089) -> ("System Status.TCP/IP"=w1088:bool)
        n442 = case shown="True" w1088 {
          tunnel: [w1094 w1098] -> w1091
          tunnel: w1090 -> [w1094 w1097]
          frame False {
          }
          frame True {
            n443 = local read "Channel"() -> (w1096:enum16{"Ch1", "Ch2", "Ch3"})
            n444 = case shown="\"Ch1\", Default" w1096 {
              tunnel: ["!channel:1" ("data in") "!channel:2" ("data in") "!channel:3" ("data in")] -> w1095
              frame "Ch1", Default {
              }
              frame "Ch2" {
              }
              frame "Ch3" {
              }
            }
            n445 = call "TcpIDFGV.vi"("Error In"=w1097, "action"=enum16{"write", "read"}."read") -> ("Error Out"=w1099:errorcluster, "connection ID out"=w1100:refnum<k5>)  [unwired: 8 in]
            n446 = call "TCP_WriteRead.vi"("error in (no error)"=w1099, "data in"=w1095, "connectin ID in"=w1100) -> ("error out"=w1098:errorcluster)  [unwired: 4 in, 2 out]
          }
        }
        n447 = call <vilib>:"Add State(s) to Queue__JKI_lib_State_Machine.vi"("State(s) in (\"\")"=w1093) -> ("States Out"=w1092:string)  [unwired: 14 in]
      }
      frame "TCP: startCam" {
        # "Send Pentero setting to AB computer\n(You can make a copy of, or modify, this frame)"
        n448 = Unbundle By Name(w1106) -> ("System Status.TCP/IP"=w1105:bool)
        n449 = case shown="True" w1105 {
          tunnel: [w1111 w1113] -> w1108
          tunnel: w1107 -> [w1111 w1112]
          frame False {
          }
          frame True {
            n450 = call "TcpIDFGV.vi"("Error In"=w1112, "action"=enum16{"write", "read"}."read") -> ("Error Out"=w1114:errorcluster, "connection ID out"=w1116:refnum<k5>)  [unwired: 8 in]
            n451 = call "TCP_WriteRead.vi"("error in (no error)"=w1114, "data in"="!focus:1", "connectin ID in"=w1116) -> ("error out"=w1113:errorcluster)  [unwired: 4 in, 2 out]
          }
        }
        n452 = call <vilib>:"Add State(s) to Queue__JKI_lib_State_Machine.vi"("State(s) in (\"\")"=w1110) -> ("States Out"=w1109:string)  [unwired: 14 in]
      }
      frame "TCP: stopCam" {
        # "Send Pentero setting to AB computer\n(You can make a copy of, or modify, this frame)"
        n453 = Unbundle By Name(w1119) -> ("System Status.TCP/IP"=w1118:bool)
        n454 = case shown="True" w1118 {
          tunnel: [w1124 w1126] -> w1121
          tunnel: w1120 -> [w1124 w1125]
          frame False {
          }
          frame True {
            n455 = call "TcpIDFGV.vi"("Error In"=w1125, "action"=enum16{"write", "read"}."read") -> ("Error Out"=w1127:errorcluster, "connection ID out"=w1129:refnum<k5>)  [unwired: 8 in]
            n456 = call "TCP_WriteRead.vi"("error in (no error)"=w1127, "data in"="!focus:0", "connectin ID in"=w1129) -> ("error out"=w1126:errorcluster)  [unwired: 4 in, 2 out]
          }
        }
        n457 = call <vilib>:"Add State(s) to Queue__JKI_lib_State_Machine.vi"("State(s) in (\"\")"=w1123) -> ("States Out"=w1122:string)  [unwired: 14 in]
      }
      frame "TCP: Close" {
        # "Close TCP connection\n()"
        n458 = Unbundle By Name(w1135) -> ("System Status.TCP/IP"=w1131:bool, "listener ID"=w1134:refnum<k5>)
        n459 = TCP Close Connection(connection ID=w1134, error in (no error)=w1133) -> (error out=w1132:errorcluster)  [unwired: 1 in, 1 out]
        n460 = case shown="True" w1131 {
          tunnel: [w1140 w1142] -> w1136
          tunnel: w1132 -> [w1140 w1141]
          frame False {
          }
          frame True {
            n461 = call "TcpIDFGV.vi"("Error In"=w1141, "action"=enum16{"write", "read"}."read") -> ("Error Out"=w1144:errorcluster, "connection ID out"=w1145:refnum<k5>)  [unwired: 8 in]
            n462 = TCP Close Connection(connection ID=w1145, error in (no error)=w1144) -> (error out=w1142:errorcluster)  [unwired: 1 in, 1 out]
          }
        }
        n463 = case shown="Error .." w1136 {
          tunnel: [w1148 w1149] -> w1137
          tunnel: w1135 -> [w1147 w1149]
          frame No Error {
            w1146 = FALSE ("System Status.TCP/IP")
            n464 = Bundle By Name(cluster=w1147, "System Status.TCP/IP"=w1146) -> (w1148:T12)
            n465 = global write "GlobalVariables.vi" "TCP connected?"(w1146) -> ()
          }
          frame Error {
          }
        }
        n466 = call <vilib>:"Add State(s) to Queue__JKI_lib_State_Machine.vi"("State(s) in (\"\")"=w1139) -> ("States Out"=w1138:string)  [unwired: 14 in]
      }
      frame "---------- Temp ----------" {
        # "Template Separator\n(You can make a copy of, or modify, this frame)"
        n467 = call <vilib>:"Add State(s) to Queue__JKI_lib_State_Machine.vi"("State(s) in (\"\")"=w1153) -> ("States Out"=w1152:string)  [unwired: 14 in]
      }
    }
    n468 = Not(x=w65) -> (.not. x?=w64:bool)
    n469 = local write "ML?"(w64) -> ()
    "ML?" <- TRUE ("main loop running?")
  }
  n470 = disable-structure "Diagram Disable Structure" shown="Disabled" {
    frame Disabled {
      w1154 = T19 {"Horizontal"=500, "Vertical"=100}  # Top Left Corner
      n471 = Control Help Window(0:w1154, 1:TRUE ("Show")) -> ()
      n472 = call <vilib>:"TDMS - File Viewer.vi"() -> ()  [unwired: 6 in, 2 out]
    }
    frame Enabled {
    }
  }
  n473 = Close File(refnum=w4, error in=w3) -> ()  [unwired: 2 out]
